vi "CRYO_MASTER.vi"() -> ()   [LabVIEW 2017]
uses:
  USBData.lvclass
  LSI218Data.lvclass
  LSI336Data.lvclass
panel:
  out "Cycle #":u32=14
  in  "Measurement Interval (s)":u32=1
  in  "Stop Button":bool
  in  "?":T1(tab)=enum."MEASUREMENT"
  in  "USB Config":T2(array[cluster]) {"terminal\n type" items=["Default"=-1, "RSE"=10083, "NRSE"=10078, "Differential"=10106, "Pseudodifferential"=12529]}
  in  "RUN identifier":string="TESTRUN"
  in  "Base Path":path=path "C:/LabVIEW/DATA/TestData/TestSeries"
  in  "InstName (USB6210/6218)":string="NIUSB"
  out "error out (USB6210/6218)":errorcluster
  out "error out (LSI336)":errorcluster
  in  "InstName (LSI336)":string="LSI336"
  in  "FileFormat (336)":string="%4.4f"
  in  "LSI336Settings(X,Y)":T3(array[cluster])=[{"LSIName"="LSi336X", "Labels"=["T1K3-1", "T1K3-2", "T3He5", "T3He8"], "SensorLocations"=[enum."T1K3-1", enum."T1K3-2", enum."T3He5", enum."T3He8"], "Active?"=TRUE, "VISA res. name"="GPIB0::1::INSTR"}, {"LSIName"="LSi336Y", "Labels"=["T3He6-1", "T3He6-2", "T3He7-1", "T3He7-2"], "SensorLocations"=[enum."T3He6-1", enum."T3He6-2", enum."T3He7-1", enum."T3He7-2"], "Active?"=TRUE, "VISA res. name"="GPIB0::2::INSTR"}, {"LSIName"="LSI218C", "Labels"=["C1", "C2", "C3", "C4", "C5", "C6", "C7", "C8"], "SensorLocations"=[enum."N.C.", enum."N.C.", enum."N.C.", enum."N.C.", enum."N.C.", enum."N.C.", enum."N.C.", enum."N.C."], "Active?"=TRUE, "VISA res. name"="GPIB0::3::INSTR"}, {"LSIName"="LSI218D", "Labels"=["D1", "D2", "D3", "D4", "D5", "D6", "D7", "D8"], "SensorLocations"=[enum."N.C.", enum."N.C.", enum."N.C.", enum."N.C.", enum."N.C.", enum."N.C.", enum."N.C.", enum."N.C."], "Active?"=TRUE, "VISA res. name"="GPIB0::5::INSTR"}, {"LSIName"="LSI218E", "Labels"=["E1", "E2", "E3", "E4", "E5", "E6", "E7", "E8"], "SensorLocations"=[enum."N.C.", enum."N.C.", enum."N.C.", enum."N.C.", enum."N.C.", enum."N.C.", enum."N.C.", enum."N.C."], "Active?"=TRUE, "VISA res. name"="GPIB0::11::INSTR"}, {"LSIName"="LSI218F", "Labels"=["F1", "F2", "F3", "F4", "F5", "F6", "F7", "F8"], "SensorLocations"=[enum."N.C.", enum."N.C.", enum."N.C.", enum."N.C.", enum."N.C.", enum."N.C.", enum."N.C.", enum."N.C."], "Active?"=TRUE, "VISA res. name"="GPIB0::8::INSTR"}]
  in  "FileFormat (218)":string="%4.4f"
  in  "InstName (LSI218)":string="LSI218"
  in  "LSI218Settings(A-F)":T3(array[cluster])=[{"LSIName"="LSI218A", "Labels"=["T3He10", "T3He1-1", "TTH3", "TTH4", "TTH1", "TTH2", "T4He1", "T1K1"], "SensorLocations"=[enum."T3He10", enum."T3He1-1", enum."TTH3", enum."TTH4", enum."TTH1", enum."TTH2", enum."T4He1", enum."T1K1"], "Active?"=TRUE, "VISA res. name"="GPIB0::7::INSTR"}, {"LSIName"="LSI218B", "Labels"=["N.C.", "N.C.", "N.C.", "N.C.", "T3He2-1", "T3He2-2", "T3He3", "T3He1-4"], "SensorLocations"=[enum."N.C.", enum."N.C.", enum."N.C.", enum."T3He1-4", enum."T3He2-1", enum."T3He2-2", enum."T3He3", enum."T3He1-4"], "Active?"=TRUE, "VISA res. name"="GPIB0::4::INSTR"}, {"LSIName"="LSI218C", "Labels"=["T4He3-1", "T4He3-2", "T4He3-3", "T4He3-4", "T4He2-1", "T4He2-2", "T4He4", "T4He5"], "SensorLocations"=[enum."T4He3-1", enum."T4He3-2", enum."T4He3-3", enum."T4He3-4", enum."T4He2-1", enum."T4He2-2", enum."T4He4", enum."T4He5"], "Active?"=TRUE, "VISA res. name"="GPIB0::3::INSTR"}, {"LSIName"="LSI218D", "Labels"=["T4He6", "T4He9", "T3He1-2", "T3He1-3", "T4He7", "T4He8", "T4He10", "T1K6"], "SensorLocations"=[enum."T4He6", enum."T4He9", enum."T3He1-2", enum."T3He1-3", enum."T4He7", enum."T4He8", enum."T4He10", enum."T1K6"], "Active?"=TRUE, "VISA res. name"="GPIB0::5::INSTR"}, {"LSIName"="LSI218E", "Labels"=["TIP1", "N.C.", "TIP2", "N.C.", "TIP3", "TIP4", "TIP5", "N.C."], "SensorLocations"=[enum."TIP1", enum."N.C.", enum."TIP2", enum."N.C.", enum."TIP3", enum."TIP4", enum."TIP5", enum."N.C."], "Active?"=TRUE, "VISA res. name"="GPIB0::11::INSTR"}, {"LSIName"="LSI218F", "Labels"=["T1K2", "T1K4", "T1K5", "T3He4", "T3He9", "TIP6", "N.C.", "N.C."], "SensorLocations"=[enum."T1K2", enum."T1K4", enum."T1K5", enum."T3He4", enum."T3He9", enum."TIP6", enum."N.C.", enum."N.C."], "Active?"=TRUE, "VISA res. name"="GPIB0::8::INSTR"}]
  out "error out (LSI218)":errorcluster
  in  "FIle suffix 4":string="Graph4"
  in  "Take Screenshot! 4":bool
  in  "FIle suffix 3":string="Graph3"
  in  "Take Screenshot! 3":bool
  in  "FIle suffix 2":string="Graph2"
  in  "Take Screenshot! 2":bool
  in  "FIle suffix 1":string="Graph1"
  in  "Take Screenshot! 1":bool
  in  "log/linear 2":bool
  in  "Tab Control 2":T4(tab)
  in  "Plot selecter (USB)\n    1      2     3     4":bool[][](array[boolean])=[[FALSE, FALSE, FALSE, FALSE], [FALSE, FALSE, FALSE, FALSE], [FALSE, FALSE, FALSE, FALSE], [FALSE, FALSE, FALSE, FALSE], [FALSE, FALSE, FALSE, FALSE]]
  out "All Labels (USB)":string[](array[string])=["Vacuum insluation"]
  out "Last Data (USB)":dbl[](array[numeric])=[1.352971810976428e-15]
  out "Time of Last Measurement (USB)":timestamp=timestamp(3682066427.35907 s since 1904-01-01)
  out "USB Status":T5(ring)=enum."Ready"
  out "Time of Last Measurement (LSI218)":timestamp=timestamp(3682066427.35907 s since 1904-01-01)
  out "LSI218 Status":T6(ring)=enum."Measuring"
  out "Last Data \nLSI218 (1)":dbl[](array[numeric])=[296.34, 296.4, 295.74, 296.27, 295.16, 295.4, 294.76, 294.96, 30.0, 0.0, 0.0, 0.0, 295.7, 296.01, 295.4, 295.83, 296.03, 296.2, 295.89, 295.9, 295.63, 295.5, 295.76, 295.69]
  out "Labels LSI218 (1)":string[](array[string])=["T3He10", "T3He1-1", "TTH3", "TTH4", "TTH1", "TTH2", "T4He1", "T1K1", "N.C.", "N.C.", "N.C.", "N.C.", "T3He2-1", "T3He2-2", "T3He3", "T3He1-4", "T4He3-1", "T4He3-2", "T4He3-3", "T4He3-4", "T4He2-1", "T4He2-2", "T4He4", "T4He5"]
  in  "Plot selecter LSI218(1)\n    1      2     3     4":bool[][](array[boolean])=[[FALSE, FALSE, TRUE, FALSE], [FALSE, FALSE, FALSE, FALSE], [FALSE, FALSE, FALSE, FALSE], [FALSE, FALSE, FALSE, FALSE], [FALSE, FALSE, FALSE, FALSE], [FALSE, FALSE, FALSE, FALSE], [FALSE, FALSE, FALSE, FALSE], [FALSE, FALSE, TRUE, FALSE], [FALSE, FALSE, TRUE, FALSE], [FALSE, FALSE, FALSE, FALSE], [FALSE, FALSE, FALSE, FALSE], [FALSE, FALSE, FALSE, FALSE], [FALSE, FALSE, FALSE, FALSE], [FALSE, FALSE, FALSE, FALSE], [FALSE, FALSE, FALSE, FALSE], [FALSE, FALSE, FALSE, FALSE], [FALSE, FALSE, FALSE, FALSE], [FALSE, FALSE, FALSE, FALSE], [FALSE, FALSE, FALSE, FALSE], [FALSE, FALSE, FALSE, FALSE], [FALSE, FALSE, FALSE, FALSE], [FALSE, FALSE, FALSE, FALSE], [FALSE, FALSE, FALSE, FALSE], [FALSE, FALSE, FALSE, FALSE]]
  out "Active?\n (1)":bool[](array[boolean])=[TRUE, TRUE, TRUE, TRUE, TRUE, TRUE, TRUE, TRUE, TRUE, TRUE, TRUE, TRUE, TRUE, TRUE, TRUE, TRUE, TRUE, TRUE, TRUE, TRUE, TRUE, TRUE, TRUE, TRUE]
  out "Labels LSI218 (2)":string[](array[string])=["T4He6", "T4He9", "T3He1-2", "T3He1-3", "T4He7", "T4He8", "T4He10", "T1K6", "TIP1", "N.C.", "TIP2", "N.C.", "TIP3", "TIP4", "TIP5", "N.C.", "T1K2", "T1K4", "T1K5", "T3He4", "T3He9", "TIP6", "N.C.", "N.C."]
  out "Active?\n(2)":bool[](array[boolean])=[TRUE, TRUE, TRUE, TRUE, TRUE, TRUE, TRUE, TRUE, TRUE, TRUE, TRUE, TRUE, TRUE, TRUE, TRUE, TRUE, TRUE, TRUE, TRUE, TRUE, TRUE, TRUE, TRUE, TRUE]
  out "Last Data \nLSI218 (2)":dbl[](array[numeric])=[295.92, 296.27, 296.59, 296.18, 295.83, 296.29, 296.2, 296.2, 296.05, 0.0, 295.46, 688.49, 295.45, 295.32, 295.49, 688.58, 296.11, 300.07, 295.58, 297.14, 293.89, 294.22, 0.433, 0.0]
  in  "Plot selecter LSI218(2)\n    1      2     3     4":bool[][](array[boolean])=[[FALSE, TRUE, FALSE, FALSE], [FALSE, TRUE, FALSE, FALSE], [FALSE, FALSE, FALSE, FALSE], [FALSE, FALSE, FALSE, FALSE], [FALSE, FALSE, FALSE, FALSE], [FALSE, FALSE, FALSE, FALSE], [FALSE, FALSE, FALSE, FALSE], [FALSE, FALSE, FALSE, FALSE], [FALSE, FALSE, FALSE, FALSE], [FALSE, FALSE, FALSE, FALSE], [FALSE, FALSE, FALSE, FALSE], [FALSE, FALSE, FALSE, FALSE], [FALSE, FALSE, FALSE, FALSE], [FALSE, FALSE, FALSE, FALSE], [FALSE, FALSE, FALSE, FALSE], [FALSE, FALSE, FALSE, FALSE], [FALSE, FALSE, FALSE, FALSE], [FALSE, FALSE, FALSE, FALSE], [FALSE, FALSE, FALSE, FALSE], [FALSE, FALSE, FALSE, FALSE], [FALSE, FALSE, FALSE, FALSE], [FALSE, FALSE, FALSE, FALSE], [FALSE, FALSE, FALSE, FALSE], [FALSE, FALSE, FALSE, FALSE]]
  in  "Plot selecter LSI336 \n     1      2     3     4":bool[][](array[boolean])=[[TRUE, TRUE, TRUE, FALSE], [TRUE, TRUE, TRUE, FALSE], [TRUE, TRUE, TRUE, FALSE], [TRUE, TRUE, TRUE, FALSE], [TRUE, TRUE, TRUE, FALSE], [TRUE, TRUE, TRUE, FALSE], [TRUE, FALSE, FALSE, FALSE], [TRUE, FALSE, FALSE, FALSE]]
  out "Time of Last Measurement (LSI336) 2":timestamp=timestamp(3682066427.35907 s since 1904-01-01)
  out "Last Data \nLSI336":dbl[](array[numeric])=[296.068, 295.808, 295.547, 295.673, 295.509, 295.453, 295.537, 295.995, 296.03, 296.03, 296.03, 296.03, 295.91, 295.91, 295.91, 295.91, 296.05, 296.05, 296.05, 296.04, 295.94, 296.19, 296.19, 296.19]
  out "Active?\n(LSI336)":bool[](array[boolean])=[TRUE, TRUE, TRUE, TRUE, TRUE, TRUE, TRUE, TRUE, TRUE, TRUE, TRUE, TRUE, TRUE, TRUE, TRUE, TRUE, TRUE, TRUE, TRUE, TRUE, TRUE, TRUE, TRUE, TRUE]
  out "Labels LSI336":string[](array[string])=["T1K3-1", "T1K3-2", "T3He5", "T3He8", "T3He6-1", "T3He6-2", "T3He7-1", "T3He7-2"]
  out "LSI336 Status":T6(ring)=enum."Measuring"
  out "Graph 1":T7(graph)=[{"TimeArray"=[timestamp(3682066413.8119783 s since 1904-01-01), timestamp(3682066414.812004 s since 1904-01-01), timestamp(3682066415.812357 s since 1904-01-01), timestamp(3682066416.9276495 s since 1904-01-01), timestamp(3682066417.9503336 s since 1904-01-01), timestamp(3682066419.060584 s since 1904-01-01), timestamp(3682066420.1444106 s since 1904-01-01), timestamp(3682066421.1446137 s since 1904-01-01), timestamp(3682066422.145889 s since 1904-01-01), timestamp(3682066423.1458697 s since 1904-01-01), timestamp(3682066424.156933 s since 1904-01-01), timestamp(3682066425.280095 s since 1904-01-01), timestamp(3682066426.3586183 s since 1904-01-01), timestamp(3682066427.35907 s since 1904-01-01)], "LDArray"=[296.065, 296.062, 296.075, 296.079, 296.076, 296.079, 296.07, 296.069, 296.077, 296.071, 296.074, 296.068, 296.073, 296.068]}, {"TimeArray"=[timestamp(3682066413.8119783 s since 1904-01-01), timestamp(3682066414.812004 s since 1904-01-01), timestamp(3682066415.812357 s since 1904-01-01), timestamp(3682066416.9276495 s since 1904-01-01), timestamp(3682066417.9503336 s since 1904-01-01), timestamp(3682066419.060584 s since 1904-01-01), timestamp(3682066420.1444106 s since 1904-01-01), timestamp(3682066421.1446137 s since 1904-01-01), timestamp(3682066422.145889 s since 1904-01-01), timestamp(3682066423.1458697 s since 1904-01-01), timestamp(3682066424.156933 s since 1904-01-01), timestamp(3682066425.280095 s since 1904-01-01), timestamp(3682066426.3586183 s since 1904-01-01), timestamp(3682066427.35907 s since 1904-01-01)], "LDArray"=[295.817, 295.815, 295.818, 295.818, 295.815, 295.816, 295.819, 295.815, 295.813, 295.821, 295.813, 295.821, 295.815, 295.808]}, {"TimeArray"=[timestamp(3682066413.8119783 s since 1904-01-01), timestamp(3682066414.812004 s since 1904-01-01), timestamp(3682066415.812357 s since 1904-01-01), timestamp(3682066416.9276495 s since 1904-01-01), timestamp(3682066417.9503336 s since 1904-01-01), timestamp(3682066419.060584 s since 1904-01-01), timestamp(3682066420.1444106 s since 1904-01-01), timestamp(3682066421.1446137 s since 1904-01-01), timestamp(3682066422.145889 s since 1904-01-01), timestamp(3682066423.1458697 s since 1904-01-01), timestamp(3682066424.156933 s since 1904-01-01), timestamp(3682066425.280095 s since 1904-01-01), timestamp(3682066426.3586183 s since 1904-01-01), timestamp(3682066427.35907 s since 1904-01-01)], "LDArray"=[295.546, 295.548, 295.546, 295.554, 295.541, 295.547, 295.533, 295.554, 295.549, 295.55, 295.555, 295.557, 295.549, 295.547]}, {"TimeArray"=[timestamp(3682066413.8119783 s since 1904-01-01), timestamp(3682066414.812004 s since 1904-01-01), timestamp(3682066415.812357 s since 1904-01-01), timestamp(3682066416.9276495 s since 1904-01-01), timestamp(3682066417.9503336 s since 1904-01-01), timestamp(3682066419.060584 s since 1904-01-01), timestamp(3682066420.1444106 s since 1904-01-01), timestamp(3682066421.1446137 s since 1904-01-01), timestamp(3682066422.145889 s since 1904-01-01), timestamp(3682066423.1458697 s since 1904-01-01), timestamp(3682066424.156933 s since 1904-01-01), timestamp(3682066425.280095 s since 1904-01-01), timestamp(3682066426.3586183 s since 1904-01-01), timestamp(3682066427.35907 s since 1904-01-01)], "LDArray"=[295.674, 295.671, 295.673, 295.667, 295.677, 295.676, 295.667, 295.67, 295.685, 295.678, 295.677, 295.669, 295.676, 295.673]}, {"TimeArray"=[timestamp(3682066413.8119783 s since 1904-01-01), timestamp(3682066414.812004 s since 1904-01-01), timestamp(3682066415.812357 s since 1904-01-01), timestamp(3682066416.9276495 s since 1904-01-01), timestamp(3682066417.9503336 s since 1904-01-01), timestamp(3682066419.060584 s since 1904-01-01), timestamp(3682066420.1444106 s since 1904-01-01), timestamp(3682066421.1446137 s since 1904-01-01), timestamp(3682066422.145889 s since 1904-01-01), timestamp(3682066423.1458697 s since 1904-01-01), timestamp(3682066424.156933 s since 1904-01-01), timestamp(3682066425.280095 s since 1904-01-01), timestamp(3682066426.3586183 s since 1904-01-01), timestamp(3682066427.35907 s since 1904-01-01)], "LDArray"=[295.497, 295.506, 295.496, 295.493, 295.508, 295.491, 295.503, 295.493, 295.509, 295.495, 295.513, 295.503, 295.494, 295.509]}, {"TimeArray"=[timestamp(3682066413.8119783 s since 1904-01-01), timestamp(3682066414.812004 s since 1904-01-01), timestamp(3682066415.812357 s since 1904-01-01), timestamp(3682066416.9276495 s since 1904-01-01), timestamp(3682066417.9503336 s since 1904-01-01), timestamp(3682066419.060584 s since 1904-01-01), timestamp(3682066420.1444106 s since 1904-01-01), timestamp(3682066421.1446137 s since 1904-01-01), timestamp(3682066422.145889 s since 1904-01-01), timestamp(3682066423.1458697 s since 1904-01-01), timestamp(3682066424.156933 s since 1904-01-01), timestamp(3682066425.280095 s since 1904-01-01), timestamp(3682066426.3586183 s since 1904-01-01), timestamp(3682066427.35907 s since 1904-01-01)], "LDArray"=[295.458, 295.464, 295.45, 295.455, 295.45, 295.46, 295.456, 295.443, 295.463, 295.456, 295.455, 295.459, 295.463, 295.453]}, {"TimeArray"=[timestamp(3682066413.8119783 s since 1904-01-01), timestamp(3682066414.812004 s since 1904-01-01), timestamp(3682066415.812357 s since 1904-01-01), timestamp(3682066416.9276495 s since 1904-01-01), timestamp(3682066417.9503336 s since 1904-01-01), timestamp(3682066419.060584 s since 1904-01-01), timestamp(3682066420.1444106 s since 1904-01-01), timestamp(3682066421.1446137 s since 1904-01-01), timestamp(3682066422.145889 s since 1904-01-01), timestamp(3682066423.1458697 s since 1904-01-01), timestamp(3682066424.156933 s since 1904-01-01), timestamp(3682066425.280095 s since 1904-01-01), timestamp(3682066426.3586183 s since 1904-01-01), timestamp(3682066427.35907 s since 1904-01-01)], "LDArray"=[295.514, 295.517, 295.528, 295.528, 295.528, 295.525, 295.535, 295.518, 295.522, 295.537, 295.527, 295.526, 295.528, 295.537]}, {"TimeArray"=[timestamp(3682066413.8119783 s since 1904-01-01), timestamp(3682066414.812004 s since 1904-01-01), timestamp(3682066415.812357 s since 1904-01-01), timestamp(3682066416.9276495 s since 1904-01-01), timestamp(3682066417.9503336 s since 1904-01-01), timestamp(3682066419.060584 s since 1904-01-01), timestamp(3682066420.1444106 s since 1904-01-01), timestamp(3682066421.1446137 s since 1904-01-01), timestamp(3682066422.145889 s since 1904-01-01), timestamp(3682066423.1458697 s since 1904-01-01), timestamp(3682066424.156933 s since 1904-01-01), timestamp(3682066425.280095 s since 1904-01-01), timestamp(3682066426.3586183 s since 1904-01-01), timestamp(3682066427.35907 s since 1904-01-01)], "LDArray"=[296.001, 296.0, 296.002, 295.989, 295.983, 295.991, 295.995, 296.007, 296.001, 295.988, 295.985, 295.986, 295.99, 295.995]}] caption="XY Graph"
  in  "log/linear 1":bool
  out "Graph 2":T8(graph)=[{"TimeArray"=[timestamp(3682066413.8119783 s since 1904-01-01), timestamp(3682066414.812004 s since 1904-01-01), timestamp(3682066415.812357 s since 1904-01-01), timestamp(3682066416.9276495 s since 1904-01-01), timestamp(3682066417.9503336 s since 1904-01-01), timestamp(3682066419.060584 s since 1904-01-01), timestamp(3682066420.1444106 s since 1904-01-01), timestamp(3682066421.1446137 s since 1904-01-01), timestamp(3682066422.145889 s since 1904-01-01), timestamp(3682066423.1458697 s since 1904-01-01), timestamp(3682066424.156933 s since 1904-01-01), timestamp(3682066425.281096 s since 1904-01-01), timestamp(3682066426.3586183 s since 1904-01-01), timestamp(3682066427.35907 s since 1904-01-01)], "DataArray"=[295.89, 295.9, 295.9, 295.91, 295.91, 295.9, 295.89, 295.88, 295.91, 295.9, 295.88, 295.95, 295.88, 295.92]}, {"TimeArray"=[timestamp(3682066413.8119783 s since 1904-01-01), timestamp(3682066414.812004 s since 1904-01-01), timestamp(3682066415.812357 s since 1904-01-01), timestamp(3682066416.9276495 s since 1904-01-01), timestamp(3682066417.9503336 s since 1904-01-01), timestamp(3682066419.060584 s since 1904-01-01), timestamp(3682066420.1444106 s since 1904-01-01), timestamp(3682066421.1446137 s since 1904-01-01), timestamp(3682066422.145889 s since 1904-01-01), timestamp(3682066423.1458697 s since 1904-01-01), timestamp(3682066424.156933 s since 1904-01-01), timestamp(3682066425.281096 s since 1904-01-01), timestamp(3682066426.3586183 s since 1904-01-01), timestamp(3682066427.35907 s since 1904-01-01)], "DataArray"=[296.27, 296.25, 296.28, 296.26, 296.28, 296.26, 296.27, 296.26, 296.26, 296.27, 296.25, 296.28, 296.29, 296.27]}, {"TimeArray"=[timestamp(3682066413.8119783 s since 1904-01-01), timestamp(3682066414.812004 s since 1904-01-01), timestamp(3682066415.812357 s since 1904-01-01), timestamp(3682066416.9276495 s since 1904-01-01), timestamp(3682066417.9503336 s since 1904-01-01), timestamp(3682066419.060584 s since 1904-01-01), timestamp(3682066420.1444106 s since 1904-01-01), timestamp(3682066421.1446137 s since 1904-01-01), timestamp(3682066422.145889 s since 1904-01-01), timestamp(3682066423.1458697 s since 1904-01-01), timestamp(3682066424.156933 s since 1904-01-01), timestamp(3682066425.280095 s since 1904-01-01), timestamp(3682066426.3586183 s since 1904-01-01), timestamp(3682066427.35907 s since 1904-01-01)], "DataArray"=[296.065, 296.062, 296.075, 296.079, 296.076, 296.079, 296.07, 296.069, 296.077, 296.071, 296.074, 296.068, 296.073, 296.068]}, {"TimeArray"=[timestamp(3682066413.8119783 s since 1904-01-01), timestamp(3682066414.812004 s since 1904-01-01), timestamp(3682066415.812357 s since 1904-01-01), timestamp(3682066416.9276495 s since 1904-01-01), timestamp(3682066417.9503336 s since 1904-01-01), timestamp(3682066419.060584 s since 1904-01-01), timestamp(3682066420.1444106 s since 1904-01-01), timestamp(3682066421.1446137 s since 1904-01-01), timestamp(3682066422.145889 s since 1904-01-01), timestamp(3682066423.1458697 s since 1904-01-01), timestamp(3682066424.156933 s since 1904-01-01), timestamp(3682066425.280095 s since 1904-01-01), timestamp(3682066426.3586183 s since 1904-01-01), timestamp(3682066427.35907 s since 1904-01-01)], "DataArray"=[295.817, 295.815, 295.818, 295.818, 295.815, 295.816, 295.819, 295.815, 295.813, 295.821, 295.813, 295.821, 295.815, 295.808]}, {"TimeArray"=[timestamp(3682066413.8119783 s since 1904-01-01), timestamp(3682066414.812004 s since 1904-01-01), timestamp(3682066415.812357 s since 1904-01-01), timestamp(3682066416.9276495 s since 1904-01-01), timestamp(3682066417.9503336 s since 1904-01-01), timestamp(3682066419.060584 s since 1904-01-01), timestamp(3682066420.1444106 s since 1904-01-01), timestamp(3682066421.1446137 s since 1904-01-01), timestamp(3682066422.145889 s since 1904-01-01), timestamp(3682066423.1458697 s since 1904-01-01), timestamp(3682066424.156933 s since 1904-01-01), timestamp(3682066425.280095 s since 1904-01-01), timestamp(3682066426.3586183 s since 1904-01-01), timestamp(3682066427.35907 s since 1904-01-01)], "DataArray"=[295.546, 295.548, 295.546, 295.554, 295.541, 295.547, 295.533, 295.554, 295.549, 295.55, 295.555, 295.557, 295.549, 295.547]}, {"TimeArray"=[timestamp(3682066413.8119783 s since 1904-01-01), timestamp(3682066414.812004 s since 1904-01-01), timestamp(3682066415.812357 s since 1904-01-01), timestamp(3682066416.9276495 s since 1904-01-01), timestamp(3682066417.9503336 s since 1904-01-01), timestamp(3682066419.060584 s since 1904-01-01), timestamp(3682066420.1444106 s since 1904-01-01), timestamp(3682066421.1446137 s since 1904-01-01), timestamp(3682066422.145889 s since 1904-01-01), timestamp(3682066423.1458697 s since 1904-01-01), timestamp(3682066424.156933 s since 1904-01-01), timestamp(3682066425.280095 s since 1904-01-01), timestamp(3682066426.3586183 s since 1904-01-01), timestamp(3682066427.35907 s since 1904-01-01)], "DataArray"=[295.674, 295.671, 295.673, 295.667, 295.677, 295.676, 295.667, 295.67, 295.685, 295.678, 295.677, 295.669, 295.676, 295.673]}, {"TimeArray"=[timestamp(3682066413.8119783 s since 1904-01-01), timestamp(3682066414.812004 s since 1904-01-01), timestamp(3682066415.812357 s since 1904-01-01), timestamp(3682066416.9276495 s since 1904-01-01), timestamp(3682066417.9503336 s since 1904-01-01), timestamp(3682066419.060584 s since 1904-01-01), timestamp(3682066420.1444106 s since 1904-01-01), timestamp(3682066421.1446137 s since 1904-01-01), timestamp(3682066422.145889 s since 1904-01-01), timestamp(3682066423.1458697 s since 1904-01-01), timestamp(3682066424.156933 s since 1904-01-01), timestamp(3682066425.280095 s since 1904-01-01), timestamp(3682066426.3586183 s since 1904-01-01), timestamp(3682066427.35907 s since 1904-01-01)], "DataArray"=[295.497, 295.506, 295.496, 295.493, 295.508, 295.491, 295.503, 295.493, 295.509, 295.495, 295.513, 295.503, 295.494, 295.509]}, {"TimeArray"=[timestamp(3682066413.8119783 s since 1904-01-01), timestamp(3682066414.812004 s since 1904-01-01), timestamp(3682066415.812357 s since 1904-01-01), timestamp(3682066416.9276495 s since 1904-01-01), timestamp(3682066417.9503336 s since 1904-01-01), timestamp(3682066419.060584 s since 1904-01-01), timestamp(3682066420.1444106 s since 1904-01-01), timestamp(3682066421.1446137 s since 1904-01-01), timestamp(3682066422.145889 s since 1904-01-01), timestamp(3682066423.1458697 s since 1904-01-01), timestamp(3682066424.156933 s since 1904-01-01), timestamp(3682066425.280095 s since 1904-01-01), timestamp(3682066426.3586183 s since 1904-01-01), timestamp(3682066427.35907 s since 1904-01-01)], "DataArray"=[295.458, 295.464, 295.45, 295.455, 295.45, 295.46, 295.456, 295.443, 295.463, 295.456, 295.455, 295.459, 295.463, 295.453]}] caption="XY Graph"
  out "Graph 3":T8(graph)=[{"TimeArray"=[timestamp(3682066413.8119783 s since 1904-01-01), timestamp(3682066414.812004 s since 1904-01-01), timestamp(3682066415.812357 s since 1904-01-01), timestamp(3682066416.9276495 s since 1904-01-01), timestamp(3682066417.9503336 s since 1904-01-01), timestamp(3682066419.060584 s since 1904-01-01), timestamp(3682066420.1444106 s since 1904-01-01), timestamp(3682066421.1446137 s since 1904-01-01), timestamp(3682066422.145889 s since 1904-01-01), timestamp(3682066423.1458697 s since 1904-01-01), timestamp(3682066424.156933 s since 1904-01-01), timestamp(3682066425.281096 s since 1904-01-01), timestamp(3682066426.3586183 s since 1904-01-01), timestamp(3682066427.35907 s since 1904-01-01)], "DataArray"=[296.35, 296.37, 296.36, 296.35, 296.33, 296.34, 296.35, 296.35, 296.34, 296.37, 296.31, 296.35, 296.33, 296.34]}, {"TimeArray"=[timestamp(3682066413.8119783 s since 1904-01-01), timestamp(3682066414.812004 s since 1904-01-01), timestamp(3682066415.812357 s since 1904-01-01), timestamp(3682066416.9276495 s since 1904-01-01), timestamp(3682066417.9503336 s since 1904-01-01), timestamp(3682066419.060584 s since 1904-01-01), timestamp(3682066420.1444106 s since 1904-01-01), timestamp(3682066421.1446137 s since 1904-01-01), timestamp(3682066422.145889 s since 1904-01-01), timestamp(3682066423.1458697 s since 1904-01-01), timestamp(3682066424.156933 s since 1904-01-01), timestamp(3682066425.281096 s since 1904-01-01), timestamp(3682066426.3586183 s since 1904-01-01), timestamp(3682066427.35907 s since 1904-01-01)], "DataArray"=[294.95, 294.95, 294.96, 294.95, 294.94, 294.95, 294.95, 294.95, 294.95, 294.95, 294.95, 294.95, 294.95, 294.96]}, {"TimeArray"=[timestamp(3682066413.8119783 s since 1904-01-01), timestamp(3682066414.812004 s since 1904-01-01), timestamp(3682066415.812357 s since 1904-01-01), timestamp(3682066416.9276495 s since 1904-01-01), timestamp(3682066417.9503336 s since 1904-01-01), timestamp(3682066419.060584 s since 1904-01-01), timestamp(3682066420.1444106 s since 1904-01-01), timestamp(3682066421.1446137 s since 1904-01-01), timestamp(3682066422.145889 s since 1904-01-01), timestamp(3682066423.1458697 s since 1904-01-01), timestamp(3682066424.156933 s since 1904-01-01), timestamp(3682066425.281096 s since 1904-01-01), timestamp(3682066426.3586183 s since 1904-01-01), timestamp(3682066427.35907 s since 1904-01-01)], "DataArray"=[30.0, 30.0, 30.0, 30.0, 30.0, 30.0, 30.0, 30.0, 30.0, 30.0, 30.0, 30.0, 30.0, 30.0]}, {"TimeArray"=[timestamp(3682066413.8119783 s since 1904-01-01), timestamp(3682066414.812004 s since 1904-01-01), timestamp(3682066415.812357 s since 1904-01-01), timestamp(3682066416.9276495 s since 1904-01-01), timestamp(3682066417.9503336 s since 1904-01-01), timestamp(3682066419.060584 s since 1904-01-01), timestamp(3682066420.1444106 s since 1904-01-01), timestamp(3682066421.1446137 s since 1904-01-01), timestamp(3682066422.145889 s since 1904-01-01), timestamp(3682066423.1458697 s since 1904-01-01), timestamp(3682066424.156933 s since 1904-01-01), timestamp(3682066425.280095 s since 1904-01-01), timestamp(3682066426.3586183 s since 1904-01-01), timestamp(3682066427.35907 s since 1904-01-01)], "DataArray"=[296.065, 296.062, 296.075, 296.079, 296.076, 296.079, 296.07, 296.069, 296.077, 296.071, 296.074, 296.068, 296.073, 296.068]}, {"TimeArray"=[timestamp(3682066413.8119783 s since 1904-01-01), timestamp(3682066414.812004 s since 1904-01-01), timestamp(3682066415.812357 s since 1904-01-01), timestamp(3682066416.9276495 s since 1904-01-01), timestamp(3682066417.9503336 s since 1904-01-01), timestamp(3682066419.060584 s since 1904-01-01), timestamp(3682066420.1444106 s since 1904-01-01), timestamp(3682066421.1446137 s since 1904-01-01), timestamp(3682066422.145889 s since 1904-01-01), timestamp(3682066423.1458697 s since 1904-01-01), timestamp(3682066424.156933 s since 1904-01-01), timestamp(3682066425.280095 s since 1904-01-01), timestamp(3682066426.3586183 s since 1904-01-01), timestamp(3682066427.35907 s since 1904-01-01)], "DataArray"=[295.817, 295.815, 295.818, 295.818, 295.815, 295.816, 295.819, 295.815, 295.813, 295.821, 295.813, 295.821, 295.815, 295.808]}, {"TimeArray"=[timestamp(3682066413.8119783 s since 1904-01-01), timestamp(3682066414.812004 s since 1904-01-01), timestamp(3682066415.812357 s since 1904-01-01), timestamp(3682066416.9276495 s since 1904-01-01), timestamp(3682066417.9503336 s since 1904-01-01), timestamp(3682066419.060584 s since 1904-01-01), timestamp(3682066420.1444106 s since 1904-01-01), timestamp(3682066421.1446137 s since 1904-01-01), timestamp(3682066422.145889 s since 1904-01-01), timestamp(3682066423.1458697 s since 1904-01-01), timestamp(3682066424.156933 s since 1904-01-01), timestamp(3682066425.280095 s since 1904-01-01), timestamp(3682066426.3586183 s since 1904-01-01), timestamp(3682066427.35907 s since 1904-01-01)], "DataArray"=[295.546, 295.548, 295.546, 295.554, 295.541, 295.547, 295.533, 295.554, 295.549, 295.55, 295.555, 295.557, 295.549, 295.547]}, {"TimeArray"=[timestamp(3682066413.8119783 s since 1904-01-01), timestamp(3682066414.812004 s since 1904-01-01), timestamp(3682066415.812357 s since 1904-01-01), timestamp(3682066416.9276495 s since 1904-01-01), timestamp(3682066417.9503336 s since 1904-01-01), timestamp(3682066419.060584 s since 1904-01-01), timestamp(3682066420.1444106 s since 1904-01-01), timestamp(3682066421.1446137 s since 1904-01-01), timestamp(3682066422.145889 s since 1904-01-01), timestamp(3682066423.1458697 s since 1904-01-01), timestamp(3682066424.156933 s since 1904-01-01), timestamp(3682066425.280095 s since 1904-01-01), timestamp(3682066426.3586183 s since 1904-01-01), timestamp(3682066427.35907 s since 1904-01-01)], "DataArray"=[295.674, 295.671, 295.673, 295.667, 295.677, 295.676, 295.667, 295.67, 295.685, 295.678, 295.677, 295.669, 295.676, 295.673]}, {"TimeArray"=[timestamp(3682066413.8119783 s since 1904-01-01), timestamp(3682066414.812004 s since 1904-01-01), timestamp(3682066415.812357 s since 1904-01-01), timestamp(3682066416.9276495 s since 1904-01-01), timestamp(3682066417.9503336 s since 1904-01-01), timestamp(3682066419.060584 s since 1904-01-01), timestamp(3682066420.1444106 s since 1904-01-01), timestamp(3682066421.1446137 s since 1904-01-01), timestamp(3682066422.145889 s since 1904-01-01), timestamp(3682066423.1458697 s since 1904-01-01), timestamp(3682066424.156933 s since 1904-01-01), timestamp(3682066425.280095 s since 1904-01-01), timestamp(3682066426.3586183 s since 1904-01-01), timestamp(3682066427.35907 s since 1904-01-01)], "DataArray"=[295.497, 295.506, 295.496, 295.493, 295.508, 295.491, 295.503, 295.493, 295.509, 295.495, 295.513, 295.503, 295.494, 295.509]}, {"TimeArray"=[timestamp(3682066413.8119783 s since 1904-01-01), timestamp(3682066414.812004 s since 1904-01-01), timestamp(3682066415.812357 s since 1904-01-01), timestamp(3682066416.9276495 s since 1904-01-01), timestamp(3682066417.9503336 s since 1904-01-01), timestamp(3682066419.060584 s since 1904-01-01), timestamp(3682066420.1444106 s since 1904-01-01), timestamp(3682066421.1446137 s since 1904-01-01), timestamp(3682066422.145889 s since 1904-01-01), timestamp(3682066423.1458697 s since 1904-01-01), timestamp(3682066424.156933 s since 1904-01-01), timestamp(3682066425.280095 s since 1904-01-01), timestamp(3682066426.3586183 s since 1904-01-01), timestamp(3682066427.35907 s since 1904-01-01)], "DataArray"=[295.458, 295.464, 295.45, 295.455, 295.45, 295.46, 295.456, 295.443, 295.463, 295.456, 295.455, 295.459, 295.463, 295.453]}] caption="XY Graph"
  out "Graph 4":T8(graph) caption="XY Graph"
  in  "log/linear 4":bool
  in  "log/linear 3":bool
  out "Series 1":string[](array[string])=["T1K3-1", "T1K3-2", "T3He5", "T3He8", "T3He6-1", "T3He6-2", "T3He7-1", "T3He7-2"]
  out "Series 2":string[](array[string])=["T4He6", "T4He9", "T1K3-1", "T1K3-2", "T3He5", "T3He8", "T3He6-1", "T3He6-2"]
  out "Series 3":string[](array[string])=["T3He10", "T1K1", "N.C.", "T1K3-1", "T1K3-2", "T3He5", "T3He8", "T3He6-1", "T3He6-2"]
  out "Series 4":string[](array[string])
  out "Plot errors":errorcluster
  out "LastMeasurementConfig (218)":T9(array[cluster])=[{"LSIName"="LSI218A", "Active?"=TRUE, "LastData"=[296.34, 296.4, 295.74, 296.27, 295.16, 295.4, 294.76, 294.96], "Labels"=["T3He10", "T3He1-1", "TTH3", "TTH4", "TTH1", "TTH2", "T4He1", "T1K1"]}, {"LSIName"="LSI218B", "Active?"=TRUE, "LastData"=[30.0, 0.0, 0.0, 0.0, 295.7, 296.01, 295.4, 295.83], "Labels"=["N.C.", "N.C.", "N.C.", "N.C.", "T3He2-1", "T3He2-2", "T3He3", "T3He1-4"]}, {"LSIName"="LSI218C", "Active?"=TRUE, "LastData"=[296.03, 296.2, 295.89, 295.9, 295.63, 295.5, 295.76, 295.69], "Labels"=["T4He3-1", "T4He3-2", "T4He3-3", "T4He3-4", "T4He2-1", "T4He2-2", "T4He4", "T4He5"]}, {"LSIName"="LSI218D", "Active?"=TRUE, "LastData"=[295.92, 296.27, 296.59, 296.18, 295.83, 296.29, 296.2, 296.2], "Labels"=["T4He6", "T4He9", "T3He1-2", "T3He1-3", "T4He7", "T4He8", "T4He10", "T1K6"]}, {"LSIName"="LSI218E", "Active?"=TRUE, "LastData"=[296.05, 0.0, 295.46, 688.49, 295.45, 295.32, 295.49, 688.58], "Labels"=["TIP1", "N.C.", "TIP2", "N.C.", "TIP3", "TIP4", "TIP5", "N.C."]}, {"LSIName"="LSI218F", "Active?"=TRUE, "LastData"=[296.11, 300.07, 295.58, 297.14, 293.89, 294.22, 0.433, 0.0], "Labels"=["T1K2", "T1K4", "T1K5", "T3He4", "T3He9", "TIP6", "N.C.", "N.C."]}]
  out "DataArrayConv (USB)":dbl[][](array[numeric])=[[1.3513338263486432e-15], [1.352562128778285e-15], [1.3521525706326738e-15], [1.3525621287783957e-15], [1.3542016022612304e-15], [1.3472475353159157e-15], [1.3484721234888237e-15], [1.348472123488879e-15], [1.3484721234889342e-15], [1.348472123488879e-15], [1.354201602261175e-15], [1.3525621287783957e-15], [1.3537915476803367e-15], [1.352971810976428e-15]]
  out "LastMeasurementConfig (336)":T9(array[cluster])=[{"LSIName"="LSi336X", "Active?"=TRUE, "LastData"=[296.068, 295.808, 295.547, 295.673], "Labels"=["T1K3-1", "T1K3-2", "T3He5", "T3He8"]}, {"LSIName"="LSi336Y", "Active?"=TRUE, "LastData"=[295.509, 295.453, 295.537, 295.995], "Labels"=["T3He6-1", "T3He6-2", "T3He7-1", "T3He7-2"]}, {"LSIName"="LSI218C", "Active?"=TRUE, "LastData"=[296.03, 296.03, 296.03, 296.03], "Labels"=["C1", "C2", "C3", "C4", "C5", "C6", "C7", "C8"]}, {"LSIName"="LSI218D", "Active?"=TRUE, "LastData"=[295.91, 295.91, 295.91, 295.91], "Labels"=["D1", "D2", "D3", "D4", "D5", "D6", "D7", "D8"]}, {"LSIName"="LSI218E", "Active?"=TRUE, "LastData"=[296.05, 296.05, 296.05, 296.04], "Labels"=["E1", "E2", "E3", "E4", "E5", "E6", "E7", "E8"]}, {"LSIName"="LSI218F", "Active?"=TRUE, "LastData"=[295.94, 296.19, 296.19, 296.19], "Labels"=["F1", "F2", "F3", "F4", "F5", "F6", "F7", "F8"]}]
  # "GLOBAL STATUS/CONTROL"
  # "Global Settings"
  # "USB6210 Settings"
  # "Space for AMI level emeters"
  # "LSI218 Settings"
  # "LSI336 Settings"
  # "Graph screenshots"
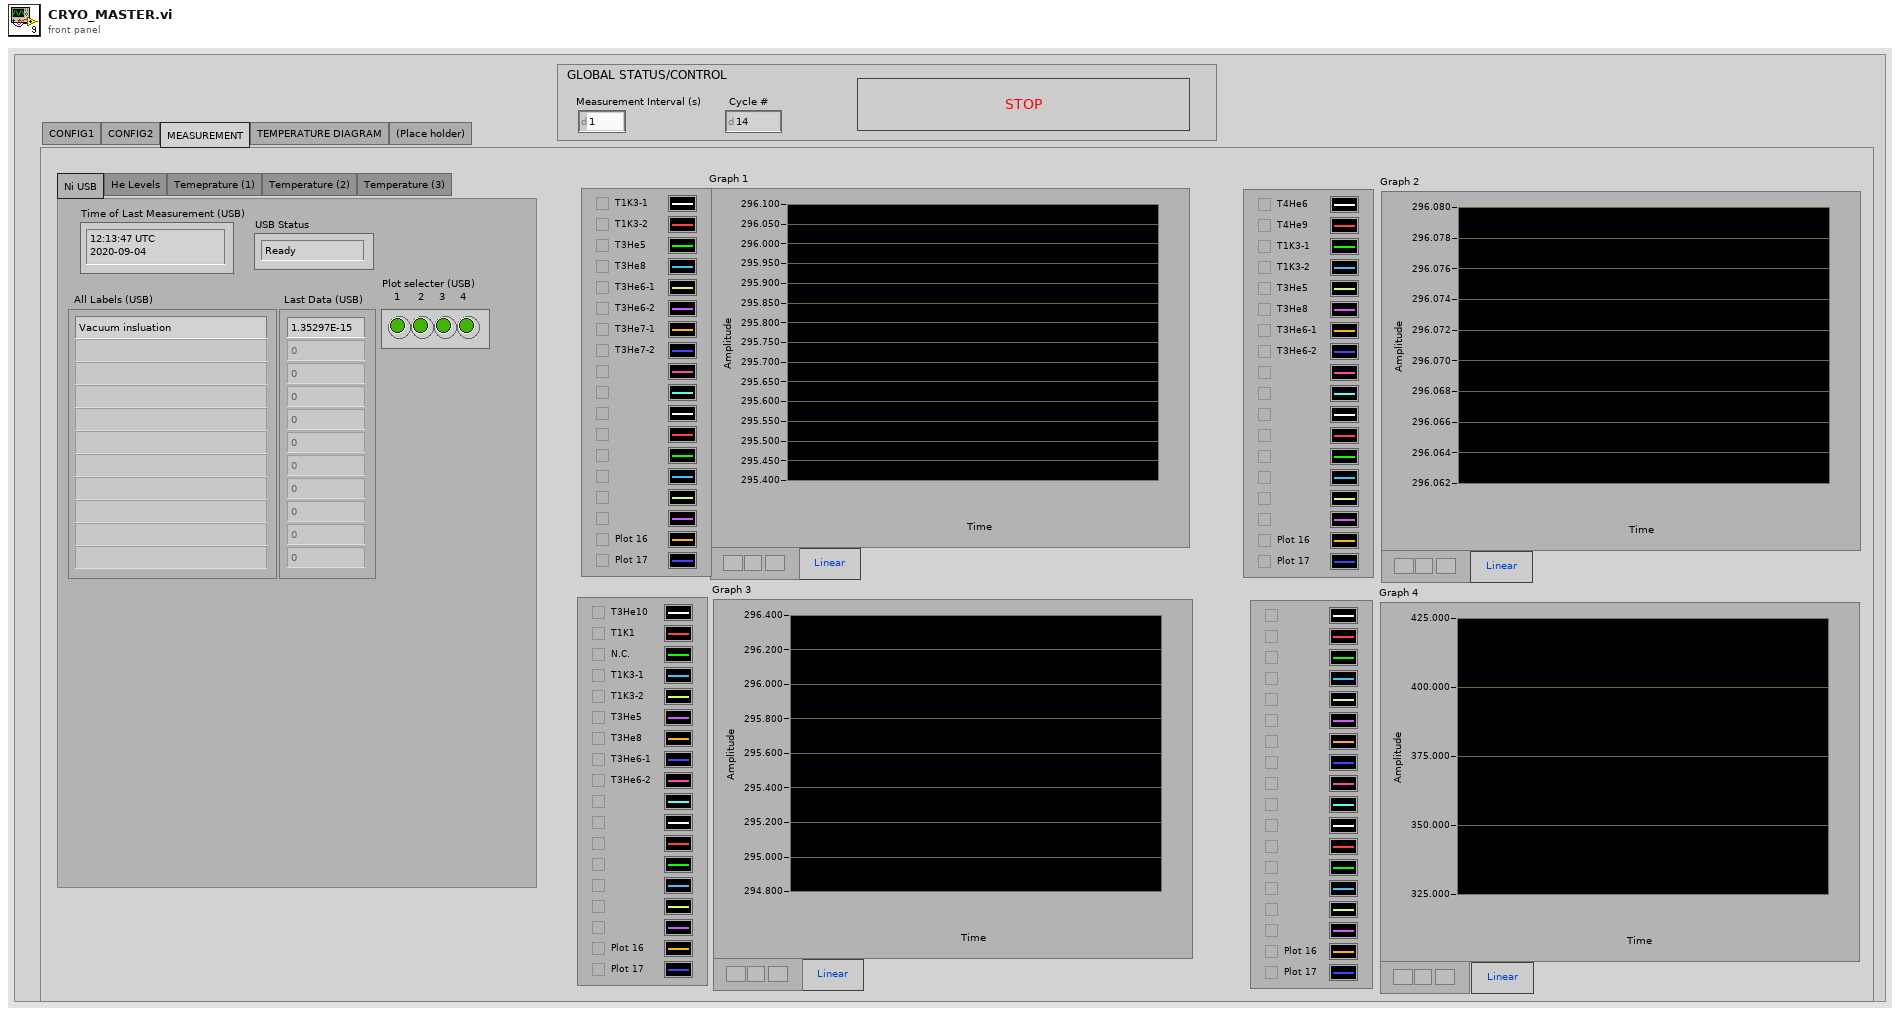
[diagram p1: front panel]
types:
  T1 = enum32{"CONFIG1", "CONFIG2", "MEASUREMENT", "TEMPERATURE DIAGRAM", "(Place holder)"}
  T2 = cluster{"Label":string, "FileFormat":string, "Active?":bool, "Physical CH":tag, " terminal\n type":i32, "ConversionType":cluster{"Type":enum16{"Raw", "SimpleProp", "CC-10_COMBINED", "CC-10_LOG", "LeakDet_EXP", "LeakDet_Mantissa", "Baratron"}, "ConversionParameters":dbl[]}, "VoltageLimits":dbl[]}[]
  T3 = cluster{"LSIName":string, "Labels":string[], "SensorLocations":enum16{"N.C.", "T3He1-1", "T3He1-2", "T3He1-3", "T3He1-4", "T3He2-1", "T3He2-2", "T3He3", "T3He4", "T3He5", "T3He6-1", "T3He6-2", "T3He7-1", "T3He7-2", "T3He8", "T3He9", "T3He10", "T4He1", "T4He2-1", "T4He2-2", "T4He3-1", "T4He3-2", "T4He3-3", "T4He3-4", "T4He4", "T4He5", "T4He6", "T4He7", "T4He8", "T4He9", "T4He10", "T1K1", "T1K2", "T1K3-1", "T1K3-2", "T1K4", "T1K5", "T1K6", "TIP1", "TIP2", "TIP3", "TIP4", "TIP5", "TIP6", "TIP7", "TTH1", "TTH2", "TTH3", "TTH4"}[], "Active?":bool, "VISA res. name":refnum<visa-resource-name>}[]
  T4 = enum32{"Ni USB", "He Levels", "Temeprature (1)", "Temperature (2)", "Temperature (3)"}
  T5 = enum16{"Intialized", "Ready", "Measuring", "Terminated"}
  T6 = enum16{"Initialized", "Ready", "Measuring", "Terminated"}
  T7 = cluster{"TimeArray":timestamp[], "LDArray":dbl[]}[]
  T8 = cluster{"TimeArray":timestamp[], "DataArray":dbl[]}[]
  T9 = cluster{"LSIName":string, "Active?":bool, "LastData":dbl[], "Labels":string[]}[]
  T10 = cluster{"TimeArray":timestamp[], "DataArrayConv":dbl[]}[]
  T11 = cluster{"IndexArray":i64[], "TimeArray":timestamp[], "DataArrayRaw":dbl[][], "DataArrayConv":dbl[][], "LDArray":dbl[]}
  T12 = cluster{"InstName":string, "Active?":bool, "Status":enum16{"Intialized", "Ready", "Measuring", "Terminated"}, "Labels":string[], "LabelLD":string, "FileFormat":string[], "FileFormatLD":string, "ReadLeakDet?":bool}
  T13 = cluster{"TimeArray":timestamp[], "DataArray":dbl[]}
  T14 = cluster{"TimeArray":timestamp[], "DataArrayConv":dbl[]}
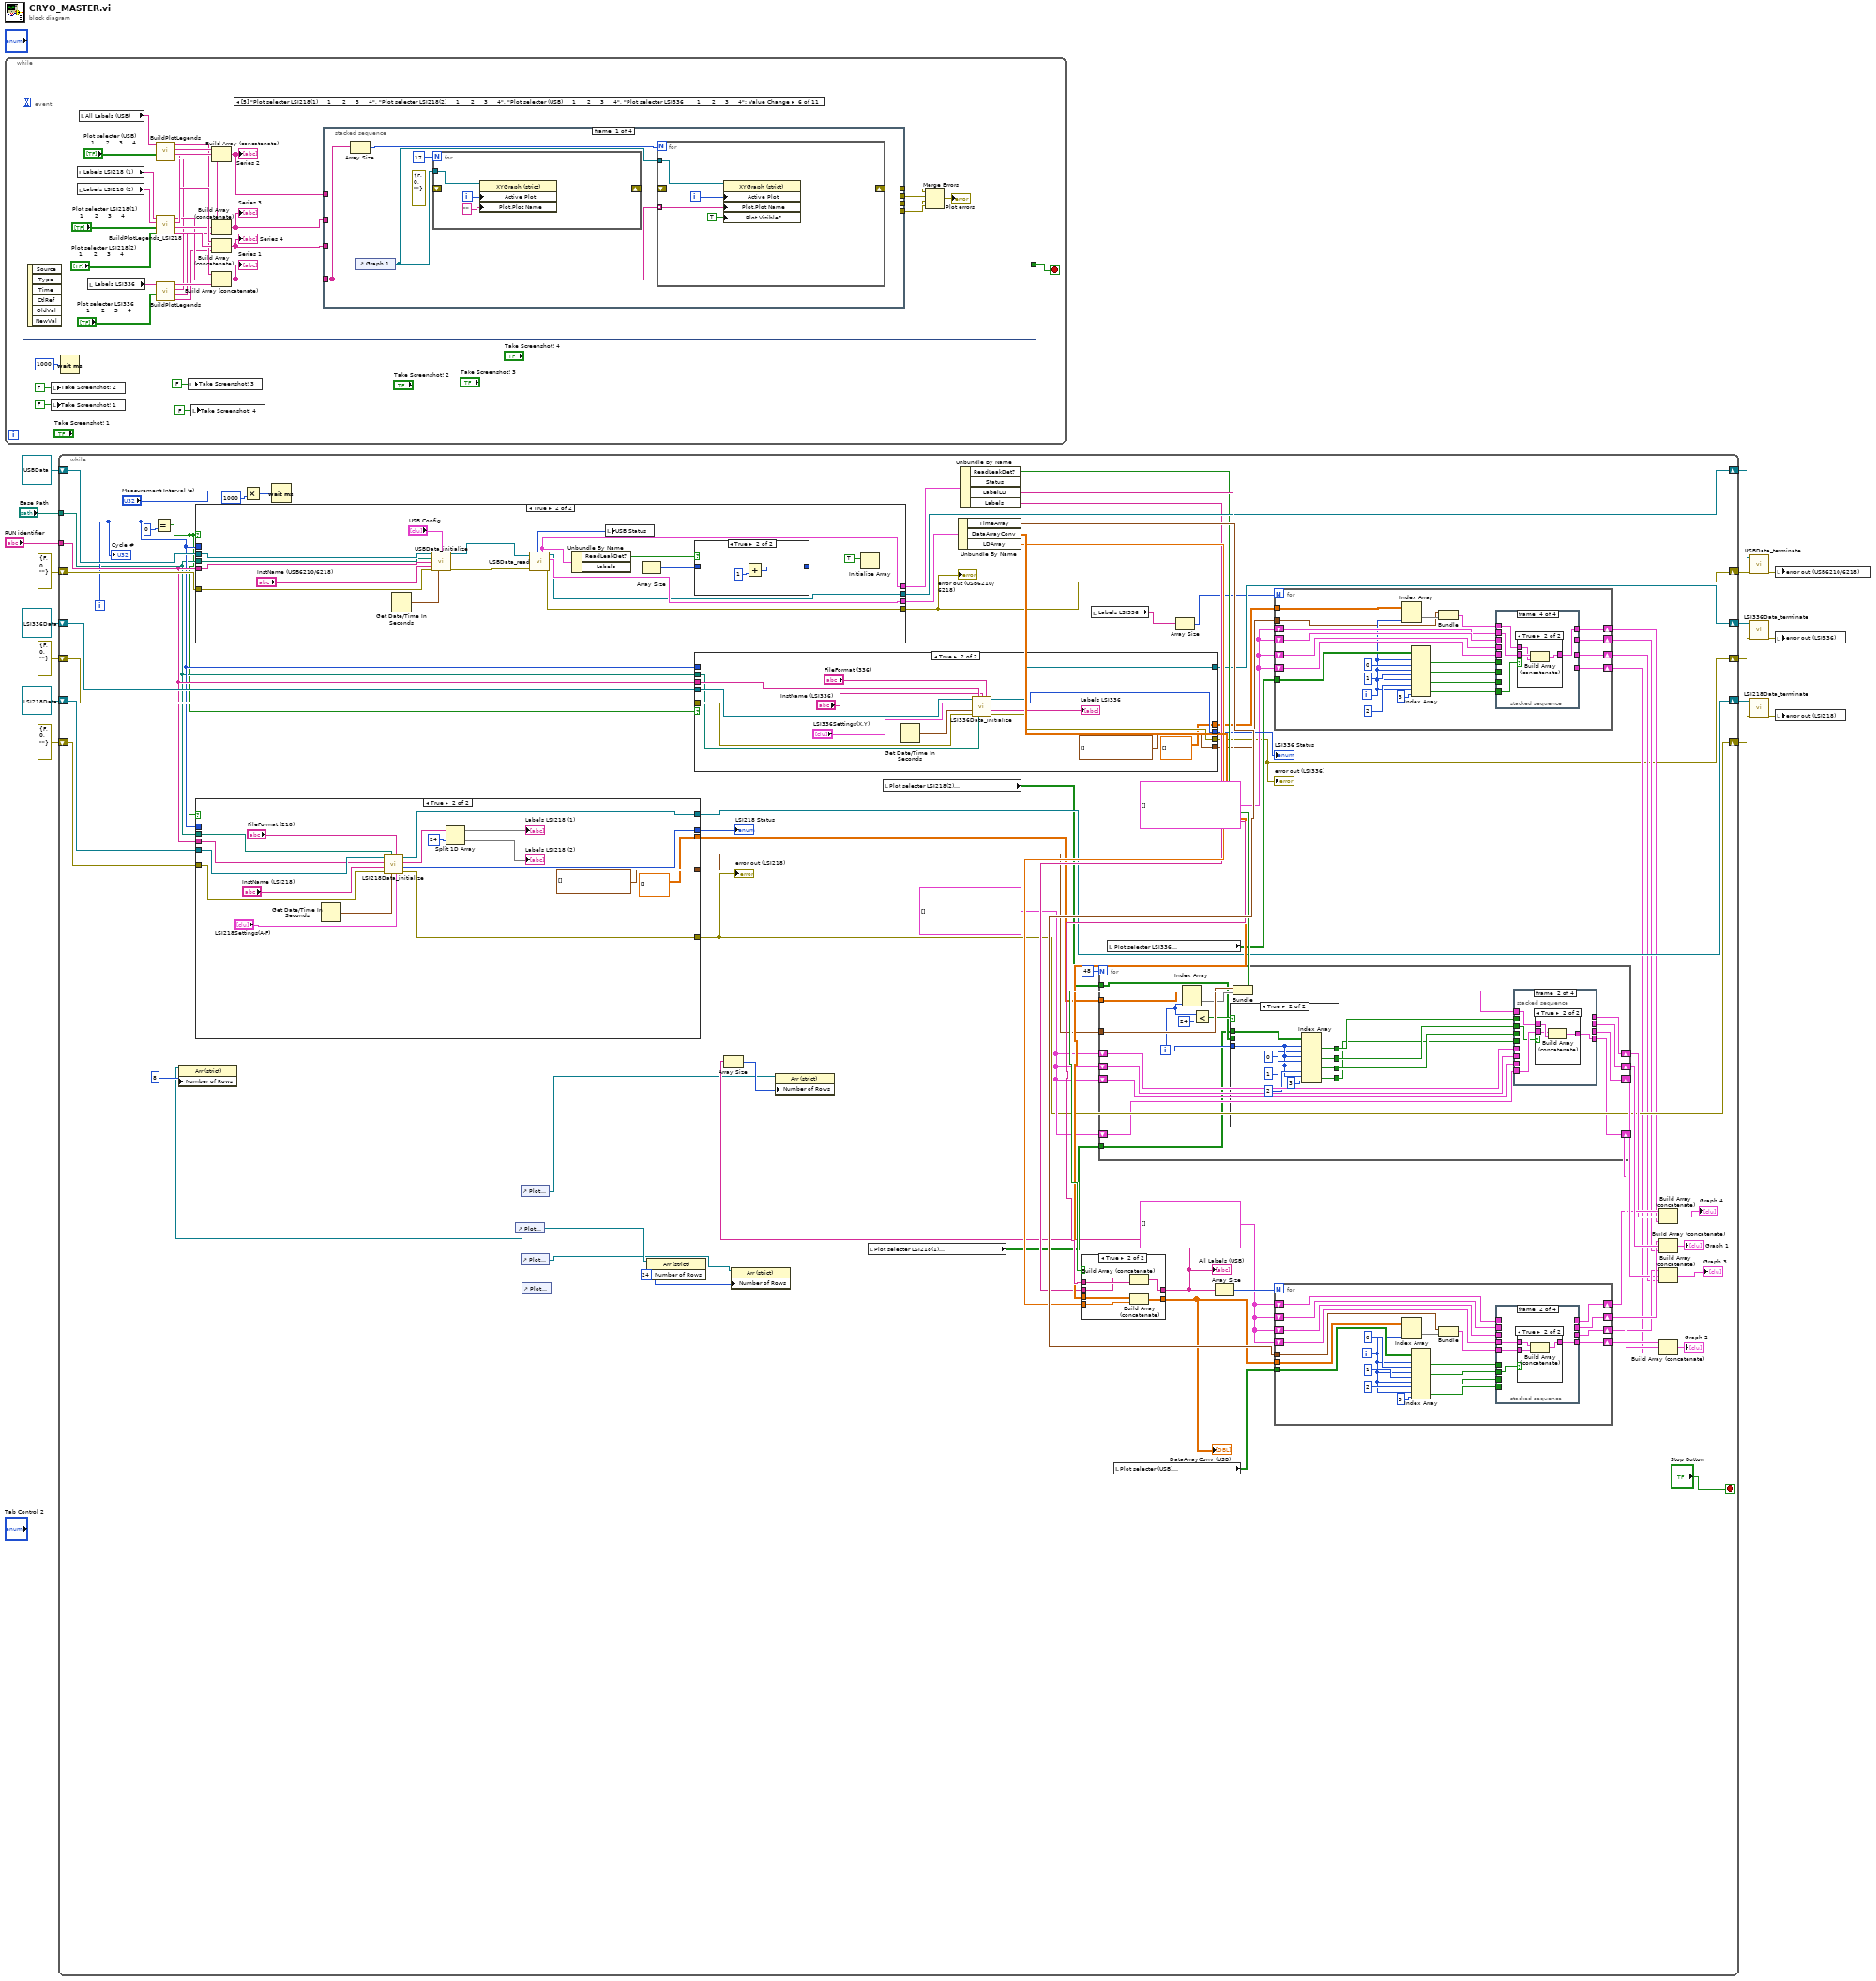
[diagram p0: block diagram]
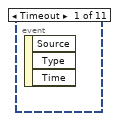
[diagram p2: hidden frame]
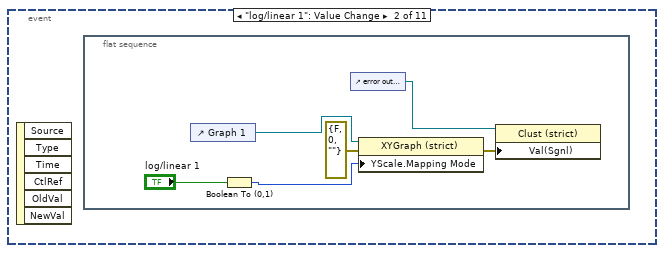
[diagram p3: hidden frame]
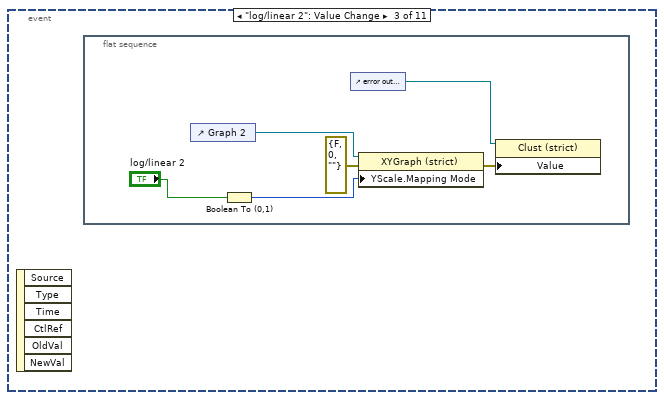
[diagram p4: hidden frame]
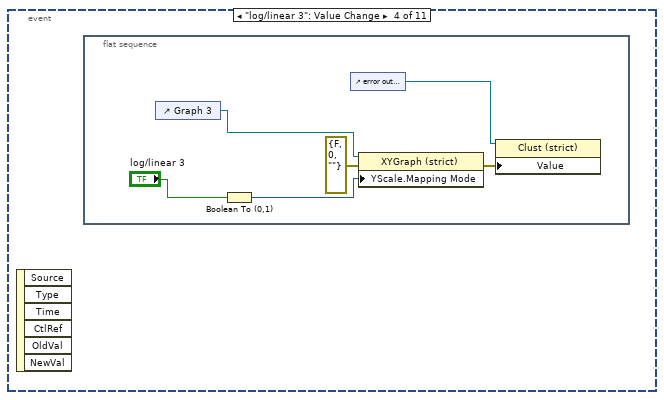
[diagram p5: hidden frame]
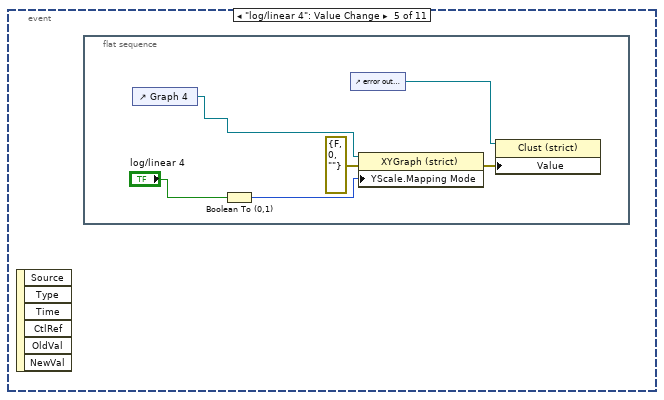
[diagram p6: hidden frame]
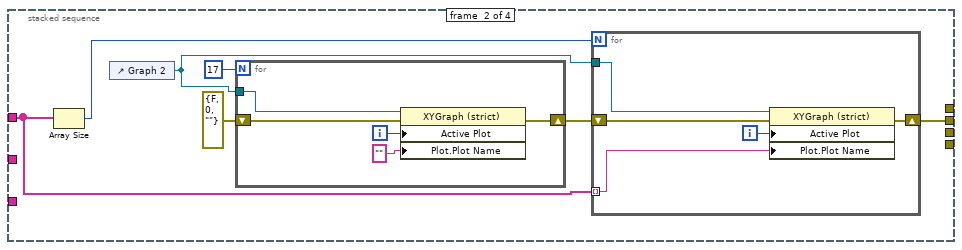
[diagram p7: hidden frame]
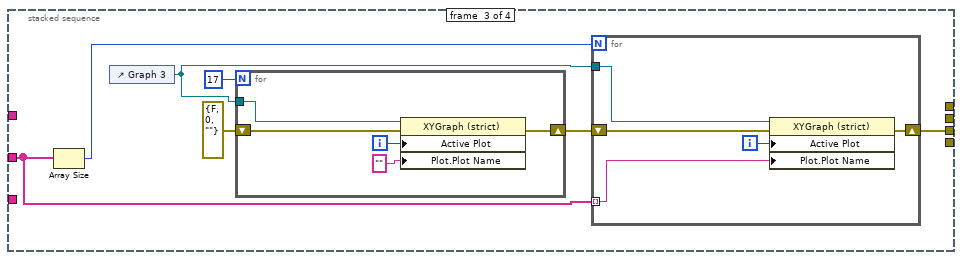
[diagram p8: hidden frame]
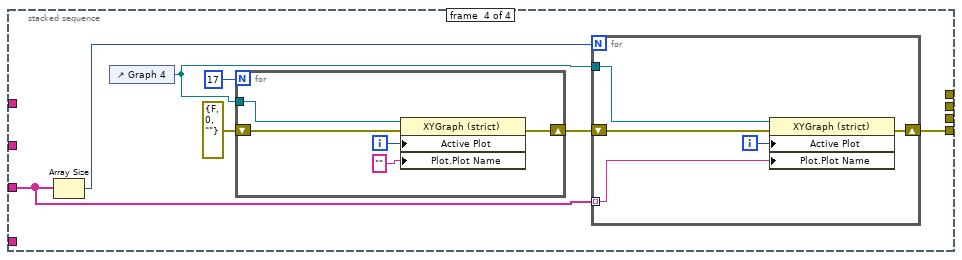
[diagram p9: hidden frame]
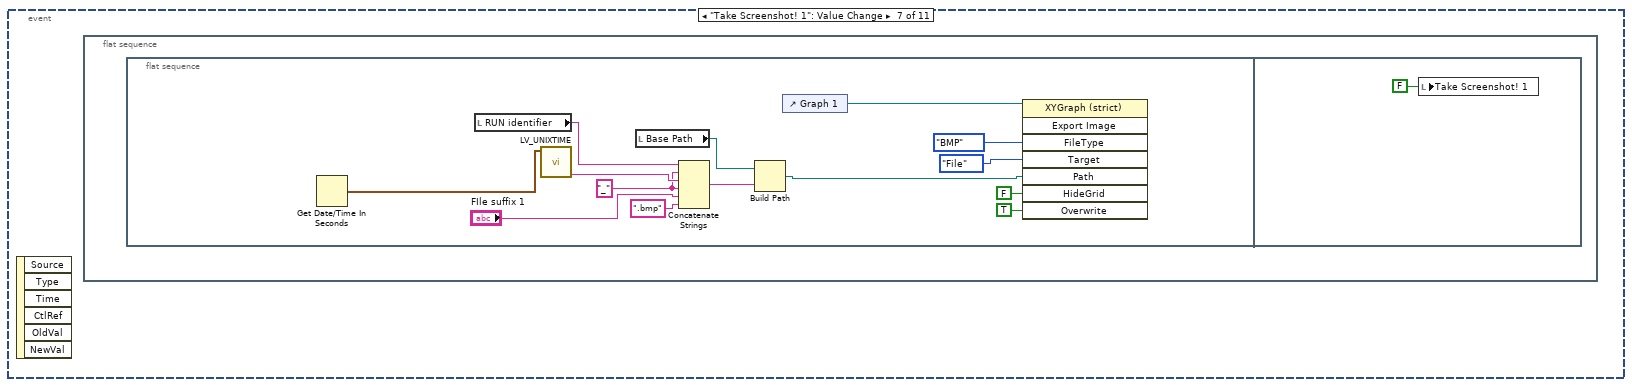
[diagram p10: hidden frame]
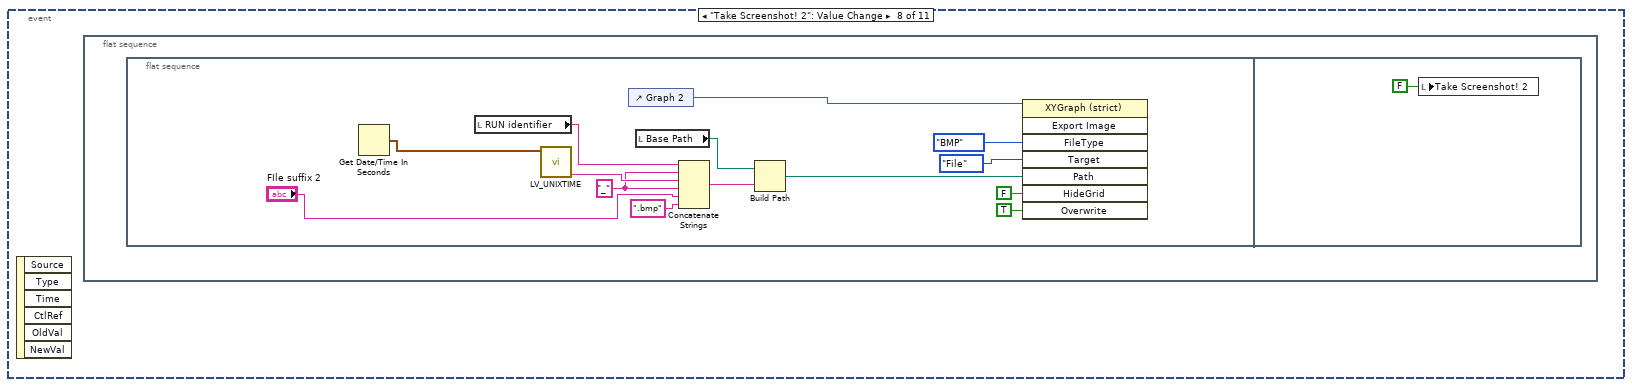
[diagram p11: hidden frame]
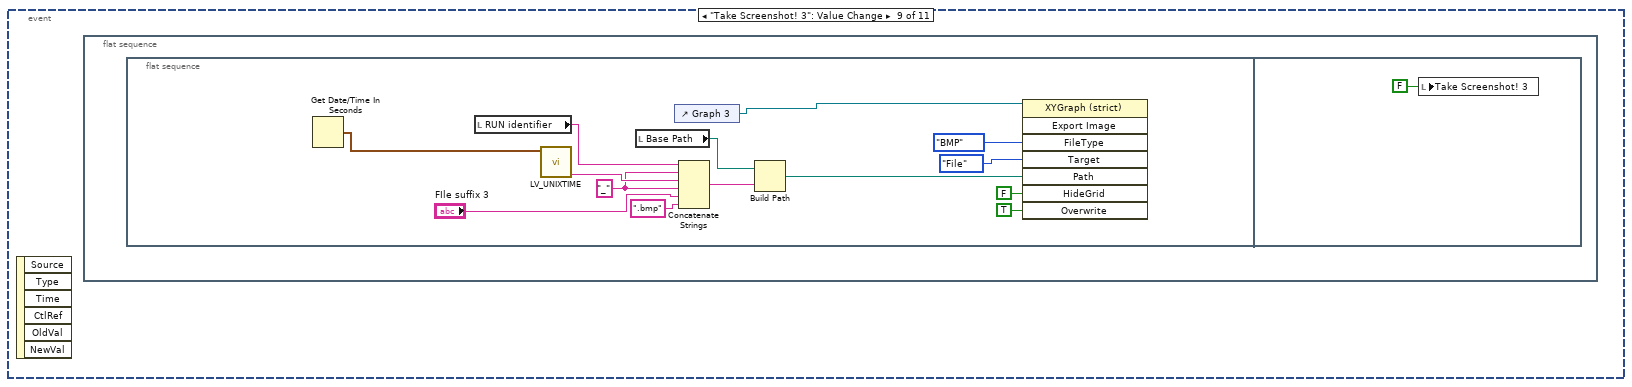
[diagram p12: hidden frame]
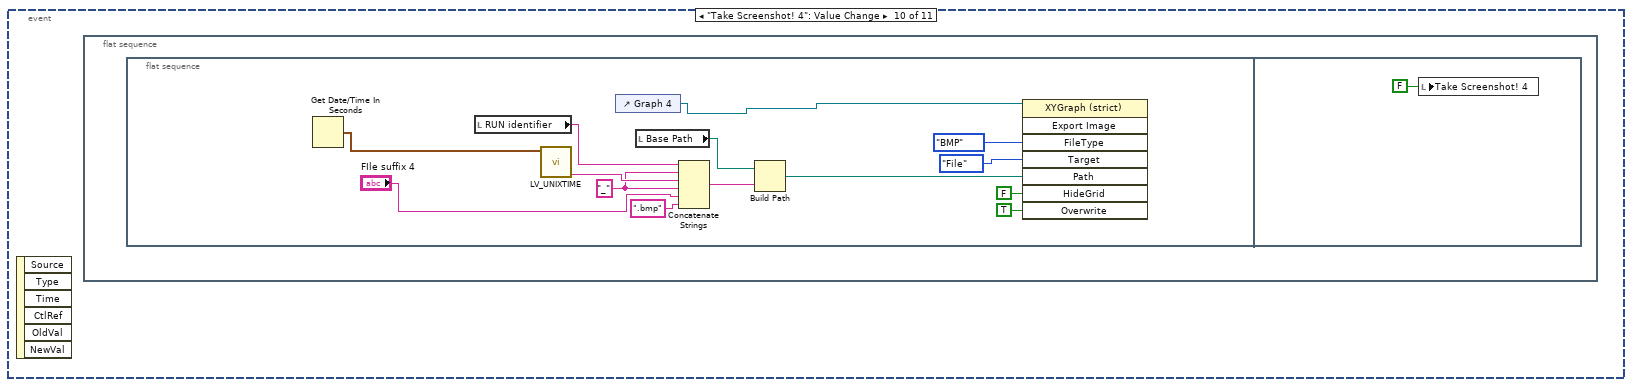
[diagram p13: hidden frame]
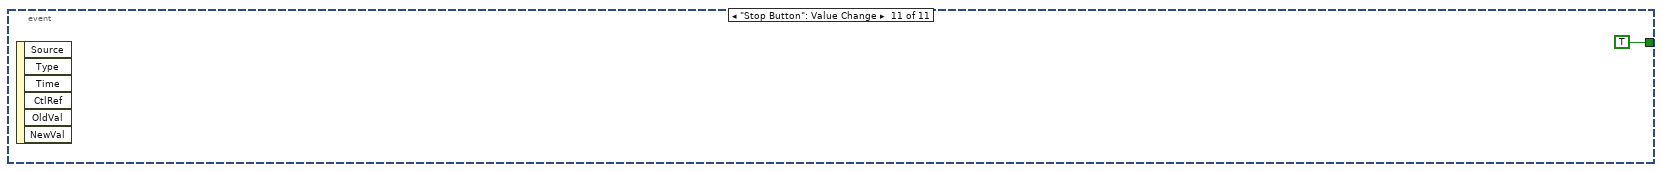
[diagram p14: hidden frame]
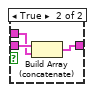
[diagram p16: hidden frame]
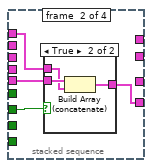
[diagram p17: hidden frame]
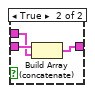
[diagram p20: hidden frame]
diagram:
  n1 = while {
    stop <- w21 stop-if-true
    n2 = event shown="[5] \"Plot selecter LSI218(1)     1      2     3     4\", \"Plot selecter LSI218(2)     1      2     3     4\", \"Plot selecter (USB)     1      2     3     4\", \"Plot selecter LSI336       1      2     3     4\": Value Change" {
      selector: _ -> [_ _ _ _ _ _ _ _ _ _ _]
      dyn-events: _ -> [_ _ _ _ _ _ _ _ _ _ _]
      timeout: _ -> [_ _ _ _ _ _ _ _ _ _ _]
      tunnel: [_ _ _ _ _ _ _ _ _ _ TRUE] -> w21
      event Timeout {
        n3 = event-data() -> ()  [unwired: 1 in, 3 out]
      }
      event "log/linear 1": Value Change {
        n4 = event-data() -> ()  [unwired: 1 in, 6 out]
        n5 = flat-sequence {
          frame #0 {
            n6 = control-ref of="Graph 1"() -> (w27:refnum<vi>)
            n7 = Boolean To (0,1)(Boolean="log/linear 1") -> (0, 1=w28:i16)
            n8 = control-ref of="error out (USB6210/6218)"() -> (w26:refnum<vi>)
            n9 = property class="XYGraph (strict)"(reference=w27, error in=errorcluster {"status"=FALSE, "code"=0, "source"=""} ("error in (no error)"), "YScale.Mapping Mode"=w28) -> (error out=w25:errorcluster)  [unwired: 1 out]
            n10 = property class="Clust (strict)"(reference=w26, "Val(Sgnl)"=w25) -> ()  [unwired: 1 in, 2 out]
          }
        }
      }
      event "log/linear 2": Value Change {
        n11 = event-data() -> ()  [unwired: 1 in, 6 out]
        n12 = flat-sequence {
          frame #0 {
            n13 = control-ref of="Graph 2"() -> (w32:refnum<vi>)
            n14 = Boolean To (0,1)(Boolean="log/linear 2") -> (0, 1=w34:i16)
            n15 = control-ref of="error out (USB6210/6218)"() -> (w31:refnum<vi>)
            n16 = property class="XYGraph (strict)"(reference=w32, error in=errorcluster {"status"=FALSE, "code"=0, "source"=""} ("error in (no error)"), "YScale.Mapping Mode"=w34) -> (error out=w33:errorcluster)  [unwired: 1 out]
            n17 = property class="Clust (strict)"(reference=w31, "Value"=w33) -> ()  [unwired: 1 in, 2 out]
          }
        }
      }
      event "log/linear 3": Value Change {
        n18 = event-data() -> ()  [unwired: 1 in, 6 out]
        n19 = flat-sequence {
          frame #0 {
            n20 = control-ref of="Graph 3"() -> (w36:refnum<vi>)
            n21 = Boolean To (0,1)(Boolean="log/linear 3") -> (0, 1=w40:i16)
            n22 = control-ref of="error out (USB6210/6218)"() -> (w38:refnum<vi>)
            n23 = property class="XYGraph (strict)"(reference=w36, error in=errorcluster {"status"=FALSE, "code"=0, "source"=""} ("error in (no error)"), "YScale.Mapping Mode"=w40) -> (error out=w39:errorcluster)  [unwired: 1 out]
            n24 = property class="Clust (strict)"(reference=w38, "Value"=w39) -> ()  [unwired: 1 in, 2 out]
          }
        }
      }
      event "log/linear 4": Value Change {
        n25 = event-data() -> ()  [unwired: 1 in, 6 out]
        n26 = flat-sequence {
          frame #0 {
            n27 = control-ref of="Graph 4"() -> (w42:refnum<vi>)
            n28 = Boolean To (0,1)(Boolean="log/linear 4") -> (0, 1=w46:i16)
            n29 = control-ref of="error out (USB6210/6218)"() -> (w44:refnum<vi>)
            n30 = property class="XYGraph (strict)"(reference=w42, error in=errorcluster {"status"=FALSE, "code"=0, "source"=""} ("error in (no error)"), "YScale.Mapping Mode"=w46) -> (error out=w45:errorcluster)  [unwired: 1 out]
            n31 = property class="Clust (strict)"(reference=w44, "Value"=w45) -> ()  [unwired: 1 in, 2 out]
          }
        }
      }
      event "Plot selecter LSI218(1)\n    1      2     3     4", "Plot selecter LSI218(2)\n    1      2     3     4", "Plot selecter (USB)\n    1      2     3     4", "Plot selecter LSI336 \n     1      2     3     4": Value Change {
        n32 = event-data() -> ()  [unwired: 1 in, 6 out]
        n33 = local read "Labels LSI218 (1)"() -> (w60:string[])
        n34 = local read "Labels LSI218 (2)"() -> (w61:string[])
        n35 = local read "All Labels (USB)"() -> (w58:string[])
        n36 = local read "Labels LSI336"() -> (w53:string[])
        n37 = call "BuildPlotLegends.vi"("Plot selecter \n    1      2     3     4"="Plot selecter (USB)\n    1      2     3     4", "AllLabels"=w58) -> ("Series 4"=w70:string[], "Series 3"=w68:string[], "Series 2"=w66:string[], "Series 1"=w64:string[])  [unwired: 6 in]
        n38 = call "BuildPlotLegends_LSI218.vi"("Plot selecter (2)\n    1      2     3     5"="Plot selecter LSI218(2)\n    1      2     3     4", "Plot selecter (1)\n    1      2     3     4"="Plot selecter LSI218(1)\n    1      2     3     4", "Labels (2)"=w61, "Labels (1)"=w60) -> ("Series 4"=w71:string[], "Series 3"=w69:string[], "Series 2"=w67:string[], "Series 1"=w65:string[])  [unwired: 4 in]
        n39 = call "BuildPlotLegends.vi"("Plot selecter \n    1      2     3     4"="Plot selecter LSI336 \n     1      2     3     4", "AllLabels"=w53) -> ("Series 4"=w48:string[], "Series 3"=w49:string[], "Series 2"=w50:string[], "Series 1"=w51:string[])  [unwired: 6 in]
        n40 = Build Array (concatenate)(w66, w67, w50) -> (w55:string[])
        "Series 2" <- w55
        n41 = Build Array (concatenate)(w68, w69, w49) -> (w56:string[])
        "Series 3" <- w56
        n42 = Build Array (concatenate)(w70, w71, w48) -> (w57:string[])
        "Series 4" <- w57
        n43 = Build Array (concatenate)(w64, w65, w51) -> (w54:string[])
        "Series 1" <- w54
        n44 = stacked-sequence {
          tunnel: [w80 _ _ _] -> w75
          tunnel: [_ w99 _ _] -> w76
          tunnel: [_ _ w115 _] -> w74
          tunnel: [_ _ _ w132] -> w73
          tunnel: w54 -> [w77 _ _ _]
          tunnel: w55 -> [_ w95 _ _]
          tunnel: w56 -> [_ _ w112 _]
          tunnel: w57 -> [_ _ _ w129]
          frame #0 {
            n45 = Array Size(array=w77) -> (size(s)=w83:i32)
            n46 = control-ref of="Graph 1"() -> (w81:refnum<vi>)
            n47 = for {
              N: 17 -> [_]
              tunnel: w81 -> [w92]
              shift-right: [w90] -> w82
              shift-left: errorcluster {"status"=FALSE, "code"=0, "source"=""} ("error in (no error)") -> [w91]
              i -> [w94]
              n48 = property class="XYGraph (strict)"(reference=w92, error in=w91, "Active Plot"=w94, "Plot.Plot Name"="") -> (error out=w90:errorcluster)  [unwired: 1 out]
            }
            n49 = for {
              N: w83 -> [_]
              tunnel: w81 -> [w88]
              shift-right: [w86] -> w80
              shift-left: w82 -> [w87]
              tunnel: w77 -> [w85] mode=indexing
              i -> [w89]
              n50 = property class="XYGraph (strict)"(reference=w88, error in=w87, "Active Plot"=w89, "Plot.Plot Name"=w85, "Plot.Visible?"=TRUE ("Plot.Visible")) -> (error out=w86:errorcluster)  [unwired: 1 out]
            }
          }
          frame #1 {
            n51 = Array Size(array=w95) -> (size(s)=w101:i32)
            n52 = control-ref of="Graph 2"() -> (w98:refnum<vi>)
            n53 = for {
              N: 17 -> [_]
              shift-right: [w108] -> w100
              shift-left: errorcluster {"status"=FALSE, "code"=0, "source"=""} ("error in (no error)") -> [w109]
              tunnel: w98 -> [w107]
              i -> [w111]
              n54 = property class="XYGraph (strict)"(reference=w107, error in=w109, "Active Plot"=w111, "Plot.Plot Name"="") -> (error out=w108:errorcluster)  [unwired: 1 out]
            }
            n55 = for {
              N: w101 -> [_]
              shift-right: [w104] -> w99
              shift-left: w100 -> [w105]
              tunnel: w95 -> [w103] mode=indexing
              tunnel: w98 -> [w102]
              i -> [w106]
              n56 = property class="XYGraph (strict)"(reference=w102, error in=w105, "Active Plot"=w106, "Plot.Plot Name"=w103) -> (error out=w104:errorcluster)  [unwired: 1 out]
            }
          }
          frame #2 {
            n57 = Array Size(array=w112) -> (size(s)=w118:i32)
            n58 = control-ref of="Graph 3"() -> (w116:refnum<vi>)
            n59 = for {
              N: 17 -> [_]
              tunnel: w116 -> [w126]
              shift-right: [w124] -> w117
              shift-left: errorcluster {"status"=FALSE, "code"=0, "source"=""} ("error in (no error)") -> [w125]
              i -> [w128]
              n60 = property class="XYGraph (strict)"(reference=w126, error in=w125, "Active Plot"=w128, "Plot.Plot Name"="") -> (error out=w124:errorcluster)  [unwired: 1 out]
            }
            n61 = for {
              N: w118 -> [_]
              tunnel: w116 -> [w122]
              shift-right: [w120] -> w115
              shift-left: w117 -> [w121]
              tunnel: w112 -> [w119] mode=indexing
              i -> [w123]
              n62 = property class="XYGraph (strict)"(reference=w122, error in=w121, "Active Plot"=w123, "Plot.Plot Name"=w119) -> (error out=w120:errorcluster)  [unwired: 1 out]
            }
          }
          frame #3 {
            n63 = Array Size(array=w129) -> (size(s)=w135:i32)
            n64 = control-ref of="Graph 4"() -> (w133:refnum<vi>)
            n65 = for {
              N: 17 -> [_]
              tunnel: w133 -> [w143]
              shift-right: [w141] -> w134
              shift-left: errorcluster {"status"=FALSE, "code"=0, "source"=""} ("error in (no error)") -> [w142]
              i -> [w145]
              n66 = property class="XYGraph (strict)"(reference=w143, error in=w142, "Active Plot"=w145, "Plot.Plot Name"="") -> (error out=w141:errorcluster)  [unwired: 1 out]
            }
            n67 = for {
              N: w135 -> [_]
              tunnel: w133 -> [w139]
              shift-right: [w137] -> w132
              shift-left: w134 -> [w138]
              tunnel: w129 -> [w136] mode=indexing
              i -> [w140]
              n68 = property class="XYGraph (strict)"(reference=w139, error in=w138, "Active Plot"=w140, "Plot.Plot Name"=w136) -> (error out=w137:errorcluster)  [unwired: 1 out]
            }
          }
        }
        n69 = Merge Errors(w75, w76, w74, w73) -> (→"Plot errors":errorcluster)
      }
      event "Take Screenshot! 1": Value Change {
        n70 = event-data() -> ()  [unwired: 1 in, 6 out]
        n71 = flat-sequence {
          frame #0 {
            n72 = flat-sequence {
              frame #0 {
                w149 = "_" ("string")
                n73 = Get Date/Time In Seconds() -> (seconds since 1Jan1904=w146:timestamp)
                n74 = local read "RUN identifier"() -> (w153:string)
                n75 = call "LV_UNIXTIME.vi"("current time"=w146) -> ("date/time string"=w150:string)  [unwired: 9 in, 1 out]
                n76 = local read "Base Path"() -> (w154:path)
                n77 = Concatenate Strings(w153, w149, w150, w149, "FIle suffix 1", ".bmp" ("string")) -> (w159:string)
                n78 = Build Path(base path=w154, name or relative path=w159) -> (appended path=w158:path)
                n79 = control-ref of="Graph 1"() -> (w151:refnum<vi>)
                n80 = invoke on="Invoke Node" class="XYGraph (strict)" method="Export Image"(reference=w151, "FileType"=enum32{"BMP", "EPS", "EMF", "PICT"}."BMP" ("File Type"), "Target"=enum32{"File", "Clipboard"}."File", "Path"=w158, "HideGrid"=FALSE ("Hide Grid"), "Overwrite"=TRUE ("Always Overwrite")) -> ()  [unwired: 2 in, 8 out]
              }
              frame #1 {
                n81 = local write "Take Screenshot! 1"(FALSE ("Take Screenshot! 1")) -> ()
              }
            }
          }
        }
      }
      event "Take Screenshot! 2": Value Change {
        n82 = event-data() -> ()  [unwired: 1 in, 6 out]
        n83 = flat-sequence {
          frame #0 {
            n84 = flat-sequence {
              frame #0 {
                w165 = "_" ("string")
                n85 = Get Date/Time In Seconds() -> (seconds since 1Jan1904=w161:timestamp)
                n86 = local read "RUN identifier"() -> (w168:string)
                n87 = call "LV_UNIXTIME.vi"("current time"=w161) -> ("date/time string"=w166:string)  [unwired: 9 in, 1 out]
                n88 = control-ref of="Graph 2"() -> (w162:refnum<vi>)
                n89 = local read "Base Path"() -> (w169:path)
                n90 = Concatenate Strings(w168, w165, w166, w165, "FIle suffix 2", ".bmp" ("string")) -> (w174:string)
                n91 = Build Path(base path=w169, name or relative path=w174) -> (appended path=w173:path)
                n92 = invoke on="Invoke Node" class="XYGraph (strict)" method="Export Image"(reference=w162, "FileType"=enum32{"BMP", "EPS", "EMF", "PICT"}."BMP" ("File Type"), "Target"=enum32{"File", "Clipboard"}."File", "Path"=w173, "HideGrid"=FALSE ("Hide Grid"), "Overwrite"=TRUE ("Always Overwrite")) -> ()  [unwired: 2 in, 8 out]
              }
              frame #1 {
                n93 = local write "Take Screenshot! 2"(FALSE ("Take Screenshot! 1")) -> ()
              }
            }
          }
        }
      }
      event "Take Screenshot! 3": Value Change {
        n94 = event-data() -> ()  [unwired: 1 in, 6 out]
        n95 = flat-sequence {
          frame #0 {
            n96 = flat-sequence {
              frame #0 {
                w180 = "_" ("string")
                n97 = Get Date/Time In Seconds() -> (seconds since 1Jan1904=w178:timestamp)
                n98 = local read "RUN identifier"() -> (w183:string)
                n99 = call "LV_UNIXTIME.vi"("current time"=w178) -> ("date/time string"=w181:string)  [unwired: 9 in, 1 out]
                n100 = local read "Base Path"() -> (w184:path)
                n101 = control-ref of="Graph 3"() -> (w176:refnum<vi>)
                n102 = Concatenate Strings(w183, w180, w181, w180, "FIle suffix 3", ".bmp" ("string")) -> (w189:string)
                n103 = Build Path(base path=w184, name or relative path=w189) -> (appended path=w188:path)
                n104 = invoke on="Invoke Node" class="XYGraph (strict)" method="Export Image"(reference=w176, "FileType"=enum32{"BMP", "EPS", "EMF", "PICT"}."BMP" ("File Type"), "Target"=enum32{"File", "Clipboard"}."File", "Path"=w188, "HideGrid"=FALSE ("Hide Grid"), "Overwrite"=TRUE ("Always Overwrite")) -> ()  [unwired: 2 in, 8 out]
              }
              frame #1 {
                n105 = local write "Take Screenshot! 3"(FALSE ("Take Screenshot! 1")) -> ()
              }
            }
          }
        }
      }
      event "Take Screenshot! 4": Value Change {
        n106 = event-data() -> ()  [unwired: 1 in, 6 out]
        n107 = flat-sequence {
          frame #0 {
            n108 = flat-sequence {
              frame #0 {
                w195 = "_" ("string")
                n109 = Get Date/Time In Seconds() -> (seconds since 1Jan1904=w193:timestamp)
                n110 = local read "RUN identifier"() -> (w198:string)
                n111 = call "LV_UNIXTIME.vi"("current time"=w193) -> ("date/time string"=w196:string)  [unwired: 9 in, 1 out]
                n112 = control-ref of="Graph 4"() -> (w191:refnum<vi>)
                n113 = local read "Base Path"() -> (w199:path)
                n114 = Concatenate Strings(w198, w195, w196, w195, "FIle suffix 4", ".bmp" ("string")) -> (w204:string)
                n115 = Build Path(base path=w199, name or relative path=w204) -> (appended path=w203:path)
                n116 = invoke on="Invoke Node" class="XYGraph (strict)" method="Export Image"(reference=w191, "FileType"=enum32{"BMP", "EPS", "EMF", "PICT"}."BMP" ("File Type"), "Target"=enum32{"File", "Clipboard"}."File", "Path"=w203, "HideGrid"=FALSE ("Hide Grid"), "Overwrite"=TRUE ("Always Overwrite")) -> ()  [unwired: 2 in, 8 out]
              }
              frame #1 {
                n117 = local write "Take Screenshot! 4"(FALSE ("Take Screenshot! 1")) -> ()
              }
            }
          }
        }
      }
      event "Stop Button": Value Change {
        n118 = event-data() -> ()  [unwired: 1 in, 6 out]
      }
    }
    n119 = local write "Take Screenshot! 2"(FALSE ("Take Screenshot! 1")) -> ()
    n120 = local write "Take Screenshot! 1"(FALSE ("Take Screenshot! 1")) -> ()
    n121 = Wait (ms)(milliseconds to wait=u32 1000) -> ()  [unwired: 1 out]
    n122 = local write "Take Screenshot! 3"(FALSE ("Take Screenshot! 1")) -> ()
    n123 = local write "Take Screenshot! 4"(FALSE ("Take Screenshot! 1")) -> ()
  }
  n124 = while {
    shift-right: [w268] -> w14
    shift-left: refnum<class "USBData.lvclass"> refnum ("USBData.lvclass") -> [w276]
    shift-right: [w259] -> w13
    shift-left: errorcluster {"status"=FALSE, "code"=0, "source"=""} ("error in (no error)") -> [w275]
    tunnel: "RUN identifier" -> [w232]
    tunnel: "Base Path" -> [w230]
    shift-right: [w238] -> w7
    shift-left: errorcluster {"status"=FALSE, "code"=0, "source"=""} ("error in (no error)") -> [w257]
    shift-right: [w239] -> w8
    shift-left: refnum<class "LSI218Data.lvclass"> refnum ("LSI218Data.lvclass") -> [w256]
    shift-right: [w220] -> w3
    shift-left: refnum<class "LSI336Data.lvclass"> refnum ("LSI336Data.lvclass") -> [w234]
    shift-right: [w219] -> w2
    shift-left: errorcluster {"status"=FALSE, "code"=0, "source"=""} ("error in (no error)") -> [w233]
    i -> [w231]
    stop <- "Stop Button" stop-if-true
    w214 = u32 24 ("Number of Rows")
    w227 = T10 [] ("appended array")
    w249 = T10 [] ("appended array")
    w250 = T10 [] ("appended array")
    n125 = Equal?(x=w231, y=0) -> (x = y?=w216:bool)
    n126 = case shown="True" w216 {
      tunnel: w276 -> [w549 w572]
      tunnel: w275 -> [w543 w570]
      tunnel: w231 -> [w531 _]
      tunnel: [w540 w567] -> w259
      tunnel: [w537 w566] -> w270
      tunnel: [w538 w565] -> w268
      tunnel: [w534 w559] -> w269
      tunnel: w232 -> [_ w557]
      tunnel: w230 -> [_ w556]
      frame False {
        n127 = call-dynamic "USBData_measure.vi"("USBData in"=w549, "DAQ sample #"=i64 5, "DAQ timeout"=100.0 ("DAQ timeout (def: 100)"), "MeasurementIndex"=w531, "error in (no error)"=w543) -> ("USBData out"=w548:refnum<class "USBData.lvclass">, "TimeMeasuremeent"=w545:timestamp, "Status"=→"USB Status":T5, "LastDataAcquired"=w542:dbl[], "error out"=w544:errorcluster)  [unwired: 4 in, 2 out]
        "Time of Last Measurement (USB)" <- w545
        n128 = call-dynamic "USBData_convert.vi"("MeasurementIndex"=w531, "error in (no error)"=w544, "LastDataAcquired"=w542, "TimeMeasuremeent"=w545, "USBData in"=w548) -> ("error out"=w541:errorcluster, "LeakDet_FULL"=w535:dbl, "LastDataConverted"=w536:dbl[], "USBData out"=w539:refnum<class "USBData.lvclass">)  [unwired: 3 in]
        n129 = call "USBData_read.vi"("USBData in"=w539, "error in (no error)"=w541) -> ("Status"=w529:T5, "USBData out"=w538:refnum<class "USBData.lvclass">, "Data"=w537:T11, "Basic"=w534:T12, "error out"=w540:errorcluster)  [unwired: 2 in, 2 out]
        n130 = Unbundle By Name(w534) -> ("ReadLeakDet?"=w533:bool)
        n131 = local write "USB Status"(w529) -> ()
        n132 = case shown="True" w533 {
          tunnel: w536 -> [w550 w553]
          tunnel: w535 -> [_ w552]
          tunnel: [w550 w551] -> w532
          frame False {
          }
          frame True {
            n133 = Build Array (concatenate)(w553, w552) -> (w551:dbl[])
          }
        }
        "Last Data (USB)" <- w532
      }
      frame True {
        n134 = Get Date/Time In Seconds() -> (seconds since 1Jan1904=w558:timestamp)
        n135 = call-dynamic "USBData_initialize.vi"("USBData in"=w572, "SeriesSetting"="USB Config", "BasePath"=w556, "RunName"=w557, "FileName"="InstName (USB6210/6218)", "error in (no error)"=w570, "RUN start time"=w558) -> ("USBData out"=w568:refnum<class "USBData.lvclass">, "error out"=w569:errorcluster)  [unwired: 4 in, 3 out]
        n136 = call "USBData_read.vi"("USBData in"=w568, "error in (no error)"=w569) -> ("Status"=w555:T5, "USBData out"=w565:refnum<class "USBData.lvclass">, "Data"=w566:T11, "Basic"=w559:T12, "error out"=w567:errorcluster)  [unwired: 2 in, 2 out]
        n137 = Unbundle By Name(w559) -> ("ReadLeakDet?"=w563:bool, "Labels"=w564:string[])
        n138 = local write "USB Status"(w555) -> ()
        n139 = Array Size(array=w564) -> (size(s)=w562:i32)
        n140 = case shown="True" w563 {
          tunnel: w562 -> [w573 w575]
          tunnel: [w573 w574] -> w560
          frame False {
          }
          frame True {
            n141 = Add(x=w575, y=1) -> (x+y=w574:i32)
          }
        }
        n142 = Initialize Array(TRUE ("Activate 2"), w560) -> ()  [unwired: 1 out]
      }
    }
    "error out (USB6210/6218)" <- w259
    n143 = case shown="True" w216 {
      tunnel: [w448 w463] -> w238
      tunnel: [w443 w462] -> w258
      tunnel: [w446 w461] -> w239
      tunnel: w231 -> [w447 _]
      tunnel: w257 -> [w437 w456]
      tunnel: w256 -> [w438 w455]
      tunnel: w232 -> [_ w454]
      tunnel: w230 -> [_ w453]
      tunnel: [w435 timestamp[] [] ("TimeArray")] -> w255
      tunnel: [w434 dbl[][] [] ("DataArray")] -> w254
      frame False {
        w441 = 24 ("index")
        n144 = call-dynamic "LSI218Data_measure.vi"("LSI218Data in"=w438, "MeasurementIndex"=w447, "error in (no error)"=w437) -> ("TimeMeasuremeent"=→"Time of Last Measurement (LSI218)":timestamp, "Active?"=w442:bool[], "LSI218Data out"=w446:refnum<class "LSI218Data.lvclass">, "LastMeasurementConfig"=→"LastMeasurementConfig (218)":T9, "LastData"=w436:dbl[], "Status"=w443:u16, "TimeArray"=w435:timestamp[], "DataArray"=w434:dbl[][], "error out"=w448:errorcluster)  [unwired: 4 in]
        n145 = Split 1D Array(array=w442, index=w441) -> (first subarray=→"Active?\n (1)":bool[], second subarray=→"Active?\n(2)":bool[])
        n146 = Split 1D Array(array=w436, index=w441) -> (first subarray=→"Last Data \nLSI218 (1)":dbl[], second subarray=→"Last Data \nLSI218 (2)":dbl[])
      }
      frame True {
        n147 = Get Date/Time In Seconds() -> (seconds since 1Jan1904=w464:timestamp)
        n148 = call-dynamic "LSI218Data_initialize.vi"("LSI218Settings(A-F)"="LSI218Settings(A-F)", "FileFormat"="FileFormat (218)", "RUN start time"=w464, "base path"=w453, "error in (no error)"=w456, "InstName"="InstName (LSI218)", "RunName"=w454, "LSI218Data in"=w455) -> ("error out"=w463:errorcluster, "Status"=w462:T6, "AllLabels"=w452:string[], "LSI218Data out"=w461:refnum<class "LSI218Data.lvclass">)
        n149 = Split 1D Array(array=w452, index=24) -> (first subarray=→"Labels LSI218 (1)":string[], second subarray=→"Labels LSI218 (2)":string[])
      }
    }
    "LSI218 Status" <- w258
    "error out (LSI218)" <- w238
    n150 = Multiply(x="Measurement Interval (s)", y=u32 1000) -> (x*y=w260:u32)
    n151 = Wait (ms)(milliseconds to wait=w260) -> ()  [unwired: 1 out]
    n152 = control-ref of="Plot selecter LSI218(1)\n    1      2     3     4"() -> (w212:refnum<vi>)
    n153 = control-ref of="Plot selecter (USB)\n    1      2     3     4"() -> (w208:refnum<vi>)
    n154 = control-ref of="Plot selecter LSI218(2)\n    1      2     3     4"() -> (w211:refnum<vi>)
    n155 = control-ref of="Plot selecter LSI336 \n     1      2     3     4"() -> (w210:refnum<vi>)
    n156 = property on="Property Node" class="Arr (strict)"(reference=w210, "Number of Rows"=u32 8) -> ()  [unwired: 1 in, 2 out]
    n157 = property on="Property Node" class="Arr (strict)"(reference=w212, "Number of Rows"=w214) -> ()  [unwired: 1 in, 2 out]
    n158 = case shown="True" w216 {
      tunnel: [w343 w355] -> w219
      tunnel: [w333 w354] -> w229
      tunnel: [w342 w353] -> w220
      tunnel: [w341 timestamp[] [] ("TimeArray")] -> w225
      tunnel: [w340 dbl[][] [] ("DataArray")] -> w226
      tunnel: w234 -> [w339 w350]
      tunnel: w233 -> [w338 w349]
      tunnel: w232 -> [_ w347]
      tunnel: w231 -> [w334 _]
      tunnel: w230 -> [_ w344]
      frame False {
        n159 = call-dynamic "LSI336Data_measure.vi"("LSI336Data in"=w339, "MeasurementIndex"=w334, "error in (no error)"=w338) -> ("Active?"=→"Active?\n(LSI336)":bool[], "TimeMeasuremeent"=→"Time of Last Measurement (LSI336) 2":timestamp, "LSI336Data out"=w342:refnum<class "LSI336Data.lvclass">, "LastData"=→"Last Data \nLSI336":dbl[], "LastMeasurementConfig"=→"LastMeasurementConfig (336)":T9, "DataArray"=w340:dbl[][], "Status"=w333:u16, "TimeArray"=w341:timestamp[], "error out"=w343:errorcluster)  [unwired: 4 in]
      }
      frame True {
        n160 = Get Date/Time In Seconds() -> (seconds since 1Jan1904=w356:timestamp)
        n161 = call-dynamic "LSI336Data_initialize.vi"("LSI336Data in"=w350, "RunName"=w347, "InstName"="InstName (LSI336)", "FileFormat"="FileFormat (336)", "LSI336Settings(X, Y)"="LSI336Settings(X,Y)", "RUN start time"=w356, "error in (no error)"=w349, "base path"=w344) -> ("LSI336Data out"=w353:refnum<class "LSI336Data.lvclass">, "Status"=w354:T6, "AllLabels"=→"Labels LSI336":string[], "error out"=w355:errorcluster)  [unwired: 4 in]
      }
    }
    "LSI336 Status" <- w229
    "error out (LSI336)" <- w219
    n162 = property on="Property Node" class="Arr (strict)"(reference=w211, "Number of Rows"=w214) -> ()  [unwired: 1 in, 2 out]
    n163 = local read "Plot selecter LSI218(1)\n    1      2     3     4"() -> (w237:bool[][])
    n164 = local read "Plot selecter LSI218(2)\n    1      2     3     4"() -> (w236:bool[][])
    n165 = Unbundle By Name(w270) -> ("TimeArray"=w274:timestamp[], "DataArrayConv"=w266:dbl[][], "LDArray"=w265:dbl[])
    n166 = Unbundle By Name(w269) -> ("ReadLeakDet?"=w267:bool, "LabelLD"=w273:string, "Labels"=w263:string[])  [unwired: 1 out]
    n167 = case shown="True" w267 {
      tunnel: w273 -> [_ w474]
      tunnel: w266 -> [w468 w473]
      tunnel: w265 -> [_ w472]
      tunnel: [w468 w471] -> w264
      tunnel: w263 -> [w467 w470]
      tunnel: [w467 w469] -> w209
      frame False {
      }
      frame True {
        n168 = Build Array (concatenate)(w470, w474) -> (w469:string[])
        n169 = Build Array (concatenate)(w473, w472) -> (w471:dbl[][])
      }
    }
    "All Labels (USB)" <- w209
    "DataArrayConv (USB)" <- w264
    n170 = Array Size(array=w209) -> (size(s)=w213:i32)
    n171 = property on="Property Node" class="Arr (strict)"(reference=w208, "Number of Rows"=w213) -> ()  [unwired: 1 in, 2 out]
    n172 = local read "Labels LSI336"() -> (w218:string[])
    n173 = for {
      N: 48 -> [_]
      tunnel: w255 -> [w377]
      tunnel: w254 -> [w374]
      tunnel: w237 -> [w358]
      tunnel: w236 -> [w359]
      shift-right: [w375] -> w253
      shift-left: w249 -> [w376]
      shift-right: [w370] -> w246
      shift-left: w249 -> [w371]
      shift-right: [w369] -> w243
      shift-left: w249 -> [w368]
      shift-right: [w367] -> w241
      shift-left: w249 -> [w366]
      i -> [w364]
      n174 = Index Array(array=w374, index (col)=w364) -> (element=w373:dbl[])  [unwired: 1 in]
      n175 = Less?(x=w364, y=24) -> (x < y?=w365:bool)
      n176 = case shown="True" w365 {
        tunnel: [w382 w400] -> w363
        tunnel: [w381 w399] -> w362
        tunnel: [w380 w397] -> w361
        tunnel: [w379 w396] -> w360
        tunnel: w358 -> [_ w395]
        tunnel: w359 -> [w389 _]
        tunnel: w364 -> [w384 w392]
        frame False {
          n177 = Subtract(x=w384, y=24) -> (x-y=w388:i32)
          n178 = Index Array(array=w389, index (row) #1=w388, index (col) #1=0 ("index (row)"), index (row) #2=w388, index (col) #2=1 ("index (row)"), index (row) #3=w388, index (col) #3=2 ("index (row)"), index (row) #4=w388, index (col) #4=3 ("index (row)")) -> (element #1=w382:bool, element #2=w381:bool, element #3=w380:bool, element #4=w379:bool)
        }
        frame True {
          n179 = Index Array(array=w395, index (row) #1=w392, index (col) #1=0 ("index (row)"), index (row) #2=w392, index (col) #2=1 ("index (row)"), index (row) #3=w392, index (col) #3=2 ("index (row)"), index (row) #4=w392, index (col) #4=3 ("index (row)")) -> (element #1=w400:bool, element #2=w399:bool, element #3=w397:bool, element #4=w396:bool)
        }
      }
      n180 = Bundle("TimeArray"=w377, "DataArray"=w373) -> (w372:T13)  [unwired: 1 in]
      n181 = stacked-sequence {
        tunnel: w376 -> [w404 _ _ _]
        tunnel: [w403 _ _ _] -> w375
        tunnel: w372 -> [w402 w412 w420 w428]
        tunnel: w371 -> [_ w411 _ _]
        tunnel: [_ w410 _ _] -> w370
        tunnel: [_ _ w419 _] -> w369
        tunnel: w368 -> [_ _ w418 _]
        tunnel: [_ _ _ w427] -> w367
        tunnel: w366 -> [_ _ _ w426]
        tunnel: w363 -> [w401 _ _ _]
        tunnel: w362 -> [_ w409 _ _]
        tunnel: w361 -> [_ _ w417 _]
        tunnel: w360 -> [_ _ _ w425]
        frame #0 {
          n182 = case shown="False" w401 {
            tunnel: w402 -> [_ w406]
            tunnel: w404 -> [w405 w408]
            tunnel: [w405 w407] -> w403
            frame False {
            }
            frame True {
              n183 = Build Array (concatenate)(w408, w406) -> (w407:T8)
            }
          }
        }
        frame #1 {
          n184 = case shown="True" w409 {
            tunnel: [w413 w416] -> w410
            tunnel: w412 -> [_ w415]
            tunnel: w411 -> [w413 w414]
            frame False {
            }
            frame True {
              n185 = Build Array (concatenate)(w414, w415) -> (w416:T8)
            }
          }
        }
        frame #2 {
          n186 = case shown="True" w417 {
            tunnel: [w421 w424] -> w419
            tunnel: w420 -> [_ w423]
            tunnel: w418 -> [w421 w422]
            frame False {
            }
            frame True {
              n187 = Build Array (concatenate)(w422, w423) -> (w424:T8)
            }
          }
        }
        frame #3 {
          n188 = case shown="True" w425 {
            tunnel: [w429 w432] -> w427
            tunnel: w428 -> [_ w431]
            tunnel: w426 -> [w429 w430]
            frame False {
            }
            frame True {
              n189 = Build Array (concatenate)(w430, w431) -> (w432:T8)
            }
          }
        }
      }
    }
    n190 = local read "Plot selecter LSI336 \n     1      2     3     4"() -> (w228:bool[][])
    n191 = local read "Plot selecter (USB)\n    1      2     3     4"() -> (w235:bool[][])
    n192 = Array Size(array=w218) -> (size(s)=w217:i32)
    n193 = Array Size(array=w209) -> (size(s)=w272:i32)
    n194 = for {
      N: w217 -> [_]
      tunnel: w228 -> [w290]
      shift-right: [w284] -> w224
      shift-left: w227 -> [w299]
      shift-right: [w280] -> w223
      shift-left: w227 -> [w297]
      shift-right: [w281] -> w222
      shift-left: w227 -> [w296]
      shift-right: [w279] -> w221
      shift-left: w227 -> [w295]
      tunnel: w226 -> [w287]
      tunnel: w225 -> [w285]
      i -> [w288]
      n195 = Index Array(array=w287, index (col)=w288) -> (element=w286:dbl[])  [unwired: 1 in]
      n196 = Index Array(array=w290, index (row) #1=w288, index (col) #1=0 ("index (row)"), index (row) #2=w288, index (col) #2=1 ("index (row)"), index (row) #3=w288, index (col) #3=2 ("index (row)"), index (row) #4=w288, index (col) #4=3 ("index (row)")) -> (element #1=w289:bool, element #2=w283:bool, element #3=w282:bool, element #4=w278:bool)
      n197 = Bundle("TimeArray"=w285, "DataArray"=w286) -> (w298:T13)  [unwired: 1 in]
      n198 = stacked-sequence {
        tunnel: w299 -> [w303 _ _ _]
        tunnel: [w302 _ _ _] -> w284
        tunnel: w298 -> [w301 w311 w319 w327]
        tunnel: w297 -> [_ w310 _ _]
        tunnel: [_ w309 _ _] -> w280
        tunnel: [_ _ w318 _] -> w281
        tunnel: w296 -> [_ _ w317 _]
        tunnel: [_ _ _ w326] -> w279
        tunnel: w295 -> [_ _ _ w325]
        tunnel: w289 -> [w300 _ _ _]
        tunnel: w283 -> [_ w308 _ _]
        tunnel: w282 -> [_ _ w316 _]
        tunnel: w278 -> [_ _ _ w324]
        frame #0 {
          n199 = case shown="False" w300 {
            tunnel: w301 -> [_ w305]
            tunnel: w303 -> [w304 w307]
            tunnel: [w304 w306] -> w302
            frame False {
            }
            frame True {
              n200 = Build Array (concatenate)(w307, w305) -> (w306:T8)
            }
          }
        }
        frame #1 {
          n201 = case shown="True" w308 {
            tunnel: [w312 w315] -> w309
            tunnel: w311 -> [_ w313]
            tunnel: w310 -> [w312 w314]
            frame False {
            }
            frame True {
              n202 = Build Array (concatenate)(w314, w313) -> (w315:T8)
            }
          }
        }
        frame #2 {
          n203 = case shown="False" w316 {
            tunnel: [w320 w323] -> w318
            tunnel: w319 -> [_ w321]
            tunnel: w317 -> [w320 w322]
            frame False {
            }
            frame True {
              n204 = Build Array (concatenate)(w322, w321) -> (w323:T8)
            }
          }
        }
        frame #3 {
          n205 = case shown="True" w324 {
            tunnel: [w328 w331] -> w326
            tunnel: w327 -> [_ w329]
            tunnel: w325 -> [w328 w330]
            frame False {
            }
            frame True {
              n206 = Build Array (concatenate)(w330, w329) -> (w331:T8)
            }
          }
        }
      }
    }
    n207 = for {
      N: w272 -> [_]
      tunnel: w264 -> [w495]
      tunnel: w274 -> [w496]
      shift-right: [w490] -> w248
      shift-left: w250 -> [w493]
      shift-right: [w488] -> w242
      shift-left: w250 -> [w491]
      shift-right: [w489] -> w251
      shift-left: w250 -> [w487]
      shift-right: [w486] -> w245
      shift-left: w250 -> [w485]
      tunnel: w235 -> [w484]
      i -> [w479]
      n208 = Index Array(array=w495, index (col)=w479) -> (element=w494:dbl[])  [unwired: 1 in]
      n209 = Index Array(array=w484, index (row) #1=w479, index (col) #1=0 ("index (row)"), index (row) #2=w479, index (col) #2=1 ("index (row)"), index (row) #3=w479, index (col) #3=2 ("index (row)"), index (row) #4=w479, index (col) #4=3 ("index (row)")) -> (element #1=w478:bool, element #2=w477:bool, element #3=w476:bool, element #4=w475:bool)
      n210 = Bundle("TimeArray"=w496, "DataArrayConv"=w494) -> (w492:T14)  [unwired: 1 in]
      n211 = stacked-sequence {
        tunnel: w478 -> [w500 _ _ _]
        tunnel: w493 -> [_ w508 _ _]
        tunnel: w476 -> [_ _ w516 _]
        tunnel: w492 -> [w497 w506 w515 w521]
        tunnel: w475 -> [_ _ _ w524]
        tunnel: w491 -> [_ _ _ w523]
        tunnel: [_ _ _ w522] -> w488
        tunnel: [_ w507 _ _] -> w490
        tunnel: [w499 _ _ _] -> w489
        tunnel: w487 -> [w498 _ _ _]
        tunnel: [_ _ w514 _] -> w486
        tunnel: w485 -> [_ _ w513 _]
        tunnel: w477 -> [_ w505 _ _]
        frame #0 {
          n212 = case shown="True" w500 {
            tunnel: [w501 w504] -> w499
            tunnel: w497 -> [_ w503]
            tunnel: w498 -> [w501 w502]
            frame False {
            }
            frame True {
              n213 = Build Array (concatenate)(w502, w503) -> (w504:T10)
            }
          }
        }
        frame #1 {
          n214 = case shown="True" w505 {
            tunnel: w508 -> [w509 w512]
            tunnel: [w509 w511] -> w507
            tunnel: w506 -> [_ w510]
            frame False {
            }
            frame True {
              n215 = Build Array (concatenate)(w512, w510) -> (w511:T10)
            }
          }
        }
        frame #2 {
          n216 = case shown="True" w516 {
            tunnel: [w517 w520] -> w514
            tunnel: w515 -> [_ w519]
            tunnel: w513 -> [w517 w518]
            frame False {
            }
            frame True {
              n217 = Build Array (concatenate)(w518, w519) -> (w520:T10)
            }
          }
        }
        frame #3 {
          n218 = case shown="True" w524 {
            tunnel: [w525 w528] -> w522
            tunnel: w521 -> [_ w527]
            tunnel: w523 -> [w525 w526]
            frame False {
            }
            frame True {
              n219 = Build Array (concatenate)(w526, w527) -> (w528:T10)
            }
          }
        }
      }
    }
    n220 = Build Array (concatenate)(w242, w241, w221) -> (→"Graph 4":T10)
    n221 = Build Array (concatenate)(w251, w253, w224) -> (→"Graph 1":T10)
    n222 = Build Array (concatenate)(w245, w243, w222) -> (→"Graph 3":T10)
    n223 = Build Array (concatenate)(w248, w246, w223) -> (→"Graph 2":T10)
    "Cycle #" <- w231
  }
  n224 = call-dynamic "USBData_terminate.vi"("error in (no error)"=w13, "USBData in"=w14) -> ("error out"=w15:errorcluster)  [unwired: 8 in, 1 out]
  n225 = call-dynamic "LSI336Data_terminate.vi"("error in (no error)"=w2, "LSI336Data in"=w3) -> ("error out"=w1:errorcluster)  [unwired: 8 in, 1 out]
  n226 = call "LSI218Data_terminate.vi"("error in (no error)"=w7, "LSI218Data in"=w8) -> ("error out"=w6:errorcluster)  [unwired: 8 in, 1 out]
  n227 = local write "error out (USB6210/6218)"(w15) -> ()
  n228 = local write "error out (LSI336)"(w1) -> ()
  n229 = local write "error out (LSI218)"(w6) -> ()
